vi "UI CMD HOLDER.vi"(8 "error in (no error)":errorcluster, 10 "VI in":refnum<vi>, 11 "Stop Event":refnum<user-event>) -> (0 "error out":errorcluster)   [LabVIEW 2020]
uses:
  PCT FGV CMD.ctl
  Popup/Popup Dialog States.ctl
  Settings/Settings.ctl
  Logging/Save Configuration.ctl
  LOG/LOG Configuration.ctl
  Message Queue/Message Cluster.ctl
  ALARM/ALARM Configuration.ctl
  Valve Control/AM Configuration.ctl
  Test Driver/Test Driver Configuration.ctl
  Test Driver/System Preset.ctl
  Test Driver/Test Type.ctl
  Report/REP Configuration.ctl
  Report/Test Setting.ctl
  MOTOR/PS Hardware Configuration.ctl
  DMM/PalmSense Hardware Configuration.ctl
  <instrlib>/PalmSens SDK for LabVIEW 5.10/PalmSens/PalmSens.lvclass
  Hiden Scanner/Scanner Hardware Configuration.ctl
  MRC/MRC Configuration.ctl
  WM Pump/Pump Hardware Configuration.ctl
  controls/PCT_UI State.ctl
  Main Menu Selector.ctl
  <vilib>/Utility/miscctls.llb/LVRowAndColumnTypeDef.ctl
  HW Message Cluster.ctl
  REF Single  Name to ref convert.vi
  Message Queue/Enqueue Message (Single).vi
  REFs Name to ref convert.vi
  Message Queue/Enqueue Message (Array).vi
  <vilib>/Utility/error.llb/Error Cluster From Error Code.vi
  <vilib>/ErrorRing/Error Ring.xnode
  Settings/Settings.lvlib
  Message Queue/Message Queue.lvlib
  Settings/Settings Dialog.vi
  User Event - Stop/User Event - Stop.lvlib
  Logging/SAVE.lvlib
  LOG/LOG.lvlib
  ALARM/QCT ALARM.lvlib
  Popup/Popup Dialog.lvlib
  Report/Report.lvlib
  Settings/HW Configuration Dialog.vi
  MOTOR/MOTOR.lvlib
  Test Driver/Test Driver.lvlib
  Motion/Motion.lvlib
  DMM/PalmSens.lvlib
  Hiden Scanner/Hiden Scanner.lvlib
  Valve Control/Valve Control.lvlib
  MRC/MRC Module.lvlib
  <vilib>/Utility/cursorutil.llb/Set Cursor (Icon Pict).vi
  WM Pump/Pump.lvlib
panel:
  # "UI CMD HOLDER"
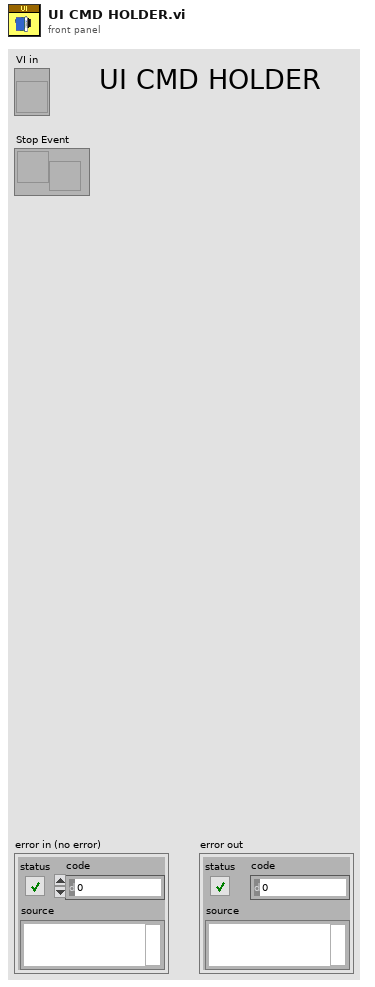
[diagram p1: front panel]
types:
  T1 = typedef "PCT FGV CMD.ctl" = enum16{"INIT", "GET", "SET"}
  T2 = typedef "Message Queue.lvlib/All Message Queues.ctl" = cluster{"UI":refnum<queue>, "Logging":refnum<queue>, "LOG":refnum<queue>, "ALARM":refnum<queue>, "Test":refnum<queue>, "Answer":refnum<queue>, "PLC":refnum<queue>, "DB":refnum<queue>, "Report":refnum<queue>, "OPC":refnum<queue>, "Procedure":refnum<queue>, "PalmSens":refnum<queue>, "SYS 7000 Reader":refnum<queue>, "SWITCH":refnum<queue>, "MOTOR":refnum<queue>, "MOTION":refnum<queue>, "HIDEN":refnum<queue>, "VALVE":refnum<queue>, "MFC":refnum<queue>, "PUMP IN":refnum<queue>, "PUMP OUT":refnum<queue>}
  T3 = typedef "PCT Data REFs.ctl" = cluster{"PLC AI Notifier":refnum<notifier>, "PS Data Queue":refnum<queue>, "BTN Queue":refnum<queue>, "PLC DI notifier":refnum<notifier>, "Timer notifier":refnum<notifier>, "DMM PS":refnum<notifier>, "DMM Gages":refnum<notifier>, "XYZ notifier":refnum<notifier>, "Test Notifier":refnum<notifier>, "Scanner notifier":refnum<notifier>, "OPC Notifier":refnum<notifier>, "HIDEN queue":refnum<queue>}
  T4 = cluster{"Type CMD":string, "Mode CMD":string, "Main CMD":string}
  T5 = typedef "Popup Dialog.lvlib/Popup Dialog States.ctl" = enum32{"Complete", "Failed", "Preparing", "Stopping", "Error", "Saved", "Saving", "Closing"}
  T6 = typedef "PCT_UI State.ctl" = enum16{"Idle", "Procedure Started", "Procedure Paused"}
  T7 = typedef "Settings.lvlib/Settings.ctl" = cluster{"Support":cluster{"Save Configuration":T8, "LOG Configuration":T9, "ALARM Configuration":T10, "User Details":string[], "Radome Type":string, "Timer Configuration":T11}, "Process":cluster{"Test Configuration":T12}, "Report Configuration":T15, "History Data":cluster{"Tests":string[][], "Test Name":string}, "Motor Configuration":T17, "PalmSense  Configuration":T18, "Hiden Scanner Resources":T19, "MFC Configuration":T20, "Pump Configuration":T21}
  T8 = typedef "SAVE.lvlib/Save Configuration.ctl" = cluster{"Log File Base Path":path, "TDMS File Reference":refnum<k34>, "Reset":bool, "Wait":dbl, "Start Time":dbl, "Update Rate":u16, "Channel Names":string[], "System Preset":variant}
  T9 = typedef "LOG.lvlib/LOG Configuration.ctl" = cluster{"LOG REF":refnum<vi>, "Writer Queue":refnum<queue>, "Log Path":path, "LOG":bool}
  T10 = typedef "QCT ALARM.lvlib/ALARM Configuration.ctl" = cluster{"LOG REF":refnum<vi>, "Writer Queue":refnum<queue>, "Log Path":path, "UPS standby":bool, "status code":i32, "SP":dbl[], "Over Sens Status":dbl[]}
  T11 = typedef "Valve Control.lvlib/AM Configuration.ctl" = cluster{"Wait":dbl, "Next Step":string, "Writer Queue":refnum<queue>, "Reset":bool, "VISA resource":refnum<visa-resource-name>, "Status":bool[], "Valve Time":dbl[], "Timer queue":refnum<queue>, "Current valve":i32, "Enable":bool}
  T12 = typedef "Test Driver.lvlib/Test Driver Configuration.ctl" = cluster{"current Step":i32, "Wait":dbl, "Next Step":string, "Writer Queue":refnum<queue>, "Reset":bool, "SEQ Time":i32, "General Reset":bool, "Cycles":i32, "Status":bool[], "Ready":bool[], "Backward":bool, "Current SP":dbl[], "System Preset":T13, "Test Type":T14, "Sample Count":i32, "Local Queues":cluster{"Cycles queue":refnum<queue>, "Step queue":refnum<queue>, "RES Queue":refnum<queue>, "Clean queue":refnum<queue>, "PS Scan queue":refnum<queue>}, "current Clean":i32, "PS Measure Plan":u16[]}
  T13 = typedef "System Preset.ctl" = cluster{"Test Configuration":cluster{"Cycles":i32, "Z Up":dbl, "SP List":dbl[][], "Operator":string, "Point Delay":i32, "Z Up 2":dbl, "Cleaning In":dbl, "Cleaning Out":dbl, "Cleaning Cycles":i32}, "Test_Start_date":string}
  T14 = typedef "Test Driver.lvlib/Test Type.ctl" = enum16{"Calibration", "Test"}
  T15 = typedef "Report.lvlib/REP Configuration.ctl" = cluster{"Test Setting":T16, "Measurements":string[][], "LOG REF":refnum<vi>, "Report Template":path, "Save Report path":path, "Data File Path":path, "Popup Dialog":bool}
  T16 = typedef "Report.lvlib/Test Setting.ctl" = cluster{"Test_Num":i32, "Test_ID":i32, "Proc_ID":i32, "Max Force":dbl, "User":string, "SN":string, "Date":string}
  T17 = typedef "MOTOR.lvlib/PS Hardware Configuration.ctl" = cluster{"Tango HW":cluster{"VISA resource":refnum<visa-resource-name>, "Baud Rate (115200)":i32, "lAnInterfaceType":i32, "bAShowProt":i32}, "Writer Queue":refnum<queue>, "Status":bool, "Abs Position":i32[], "Axis Velocity":cluster{"dX":dbl, "dY":dbl, "dZ":dbl, "dA":dbl}, "acceleration ":dbl, "Z direction":enum16{"Up", "Down"}, "Position Mode":string, "plLSID":i32}
  T18 = typedef "PalmSens.lvlib/PalmSense Hardware Configuration.ctl" = cluster{"PalmSens.lvclass":refnum<class "PalmSens.lvclass">, "Writer Queue":refnum<queue>, "Enable":bool, "Is Measuring Ref":refnum<vi>, "Method":cluster{"Name":string, "Method Ref":variant}, "PS Live Curve Result":refnum<vi>}
  T19 = typedef "Hiden Scanner.lvlib/Scanner Hardware Configuration.ctl" = cluster{"Link":cluster{"Connection":enum16{"Serial", "TCP/IP", "USB"}, "Host or IP address (TCP/IP)":string, "Port (Serial/USB)":string}, "VISA resource":refnum<visa-resource-name>, "Writer Queue":refnum<queue>, "Status":bool}
  T20 = typedef "MRC Module.lvlib/MRC Configuration.ctl" = cluster{"MFC Definition":cluster{"MFC Port":refnum<visa-resource-name>, "MFC Enable":bool, "Baud Rate":i32, "Interface type":enum32{"RS-485", "RS-232"}, "Address":i32}, "Set Point Options":cluster{"Setpoint Value":dbl, "Mass Flow EU 2":string, "Setpoint Source":string, "Valve Mode":string}, "Writer Queue":refnum<queue>, "Enable":bool, "Update Rate":u32, "MRC Chamber Enable":bool, "Selected Gas":string, "Address String":string}
  T21 = typedef "Pump.lvlib/Pump Hardware Configuration.ctl" = cluster{"Pump  name":refnum<visa-resource-name>[], "Writer Queue":refnum<queue>, "Pump Info":cluster{"Pump Type":string, "Speed":i32, "Direction":u16, "Running":bool}, "Current Pump Name":refnum<visa-resource-name>, "Wait":dbl, "Next Step":string, "Reset":bool}
  T22 = enum16{"open", "open or create", "create or replace", "create", "open (read-only)"}
  T23 = typedef "Main Menu Selector.ctl" = enum16{"Main Screen", "Test Setting", "Calibration", "History", "Admin", "Switch User", "About", "Exit"}
  T24 = cluster{"Back-Front Switch":bool, "NewVal":enum32{"1", "2", "3", "4", "5", "6", "7", "8", "9", "10", "11", "12", "13", "14", "15", "16", "17", "18", "19", "20"}}
  T25 = cluster{"Writer Queue":refnum<queue>, "Timeout":dbl[], "Status":bool[]}
  T26 = enum16{"isDO_Section_0", "isDO_Section_90", "isDO_Section_180", "isDO_Section_270", "Mode", "Start", "Reset_Error", "Heart_Beat", "Polling_Cylinder", "Turning_Cylinder", "Locking_Cylinder"}
  T27 = cluster{"Channels":enum16{"isDO_Section_0", "isDO_Section_90", "isDO_Section_180", "isDO_Section_270", "Mode", "Start", "Reset_Error", "Heart_Beat", "Polling_Cylinder", "Turning_Cylinder", "Locking_Cylinder"}, "Status":bool}
  T28 = cluster{"register":dbl, "register":dbl, "register":dbl, "register":dbl}[]
  T29 = typedef "Message Queue.lvlib/Message Cluster.ctl" = cluster{"Message":string, "Message Data":variant}
  T30 = typedef "LVRowAndColumnTypeDef.ctl" = cluster{"Row":i32, "Column":i32}
  T31 = typedef "Message Queue.lvlib/HW Message Cluster.ctl" = cluster{"Writer Queue":refnum<queue>, "Writer Data":T29}
  T32 = enum32{"1", "2", "3", "4", "5", "6", "7", "8", "9", "10", "11", "12", "13", "14", "15", "16", "17", "18", "19", "20"}
  T33 = cluster{"Pump Type":string, "Speed":i32, "Direction":u16, "Running":bool}
  T34 = cluster{"Current SP[0]":dbl, "Current SP[1]":dbl}
  T35 = cluster{"Current SP[0]":i32, "Current SP[1]":i32}
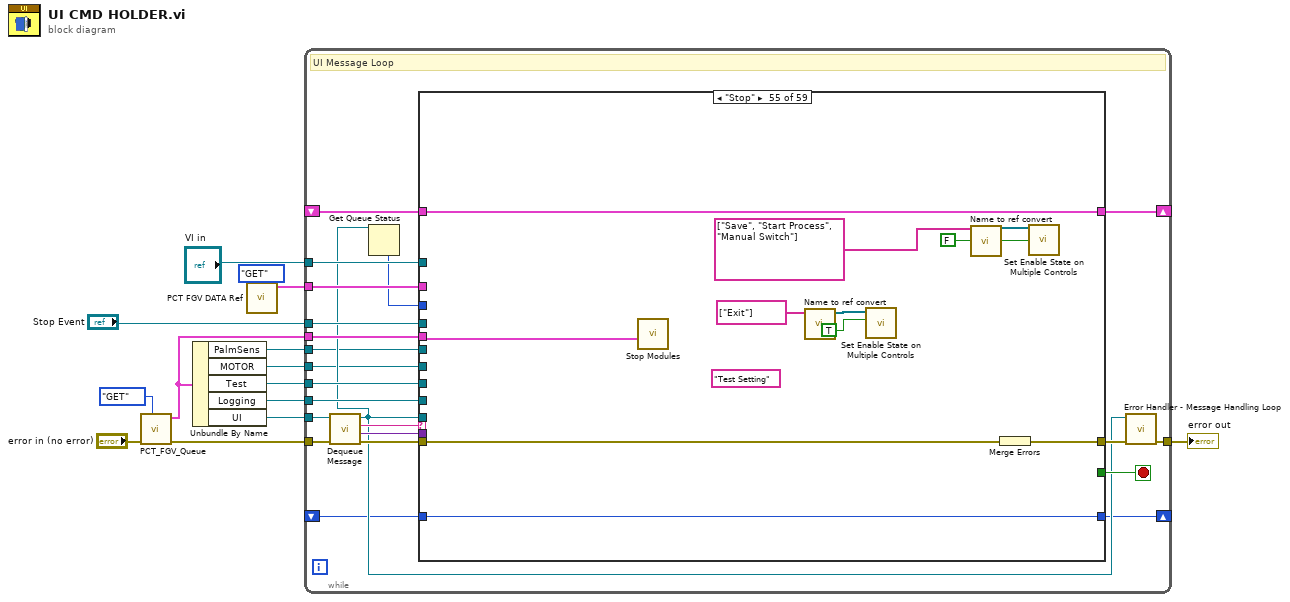
[diagram p0: block diagram]
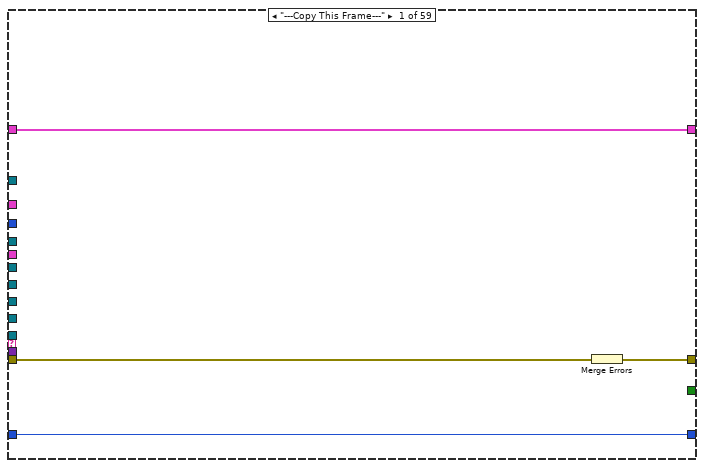
[diagram p2: hidden frame]
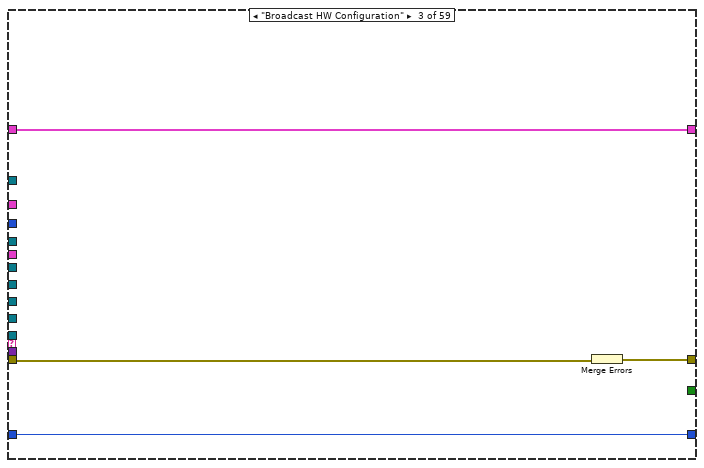
[diagram p4: hidden frame]
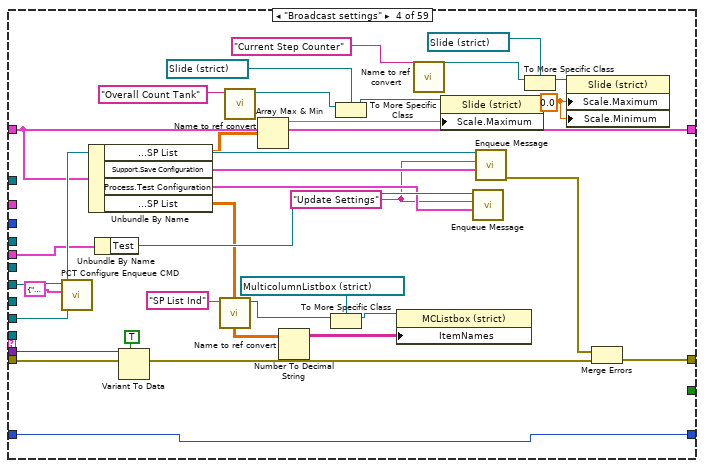
[diagram p5: hidden frame]
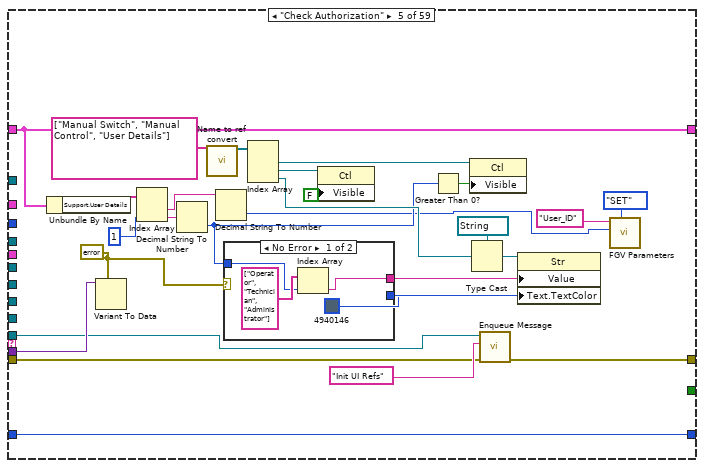
[diagram p6: hidden frame]
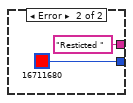
[diagram p7: hidden frame]
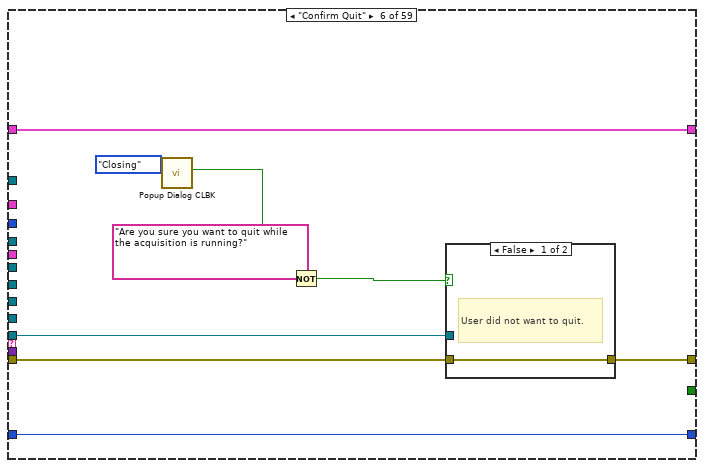
[diagram p8: hidden frame]
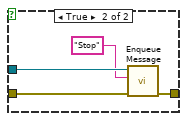
[diagram p9: hidden frame]
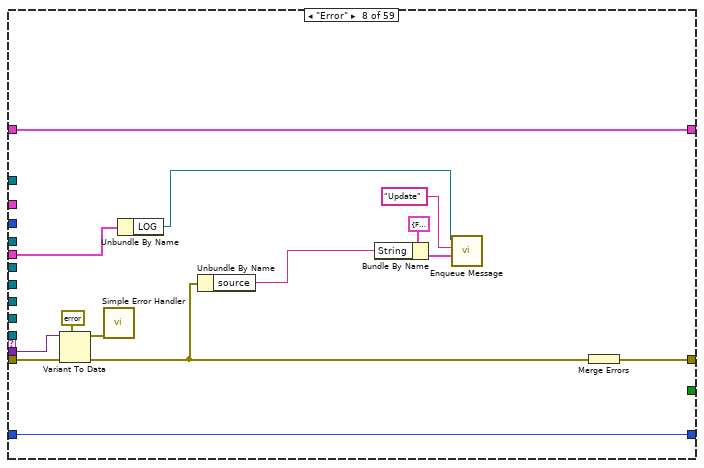
[diagram p11: hidden frame]
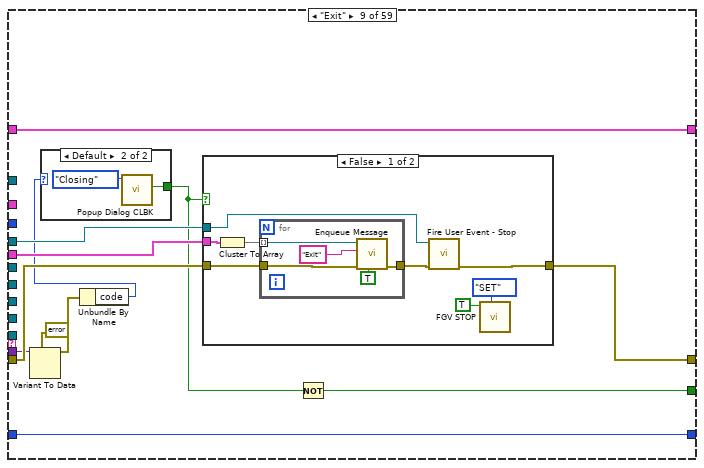
[diagram p12: hidden frame]
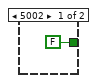
[diagram p13: hidden frame]
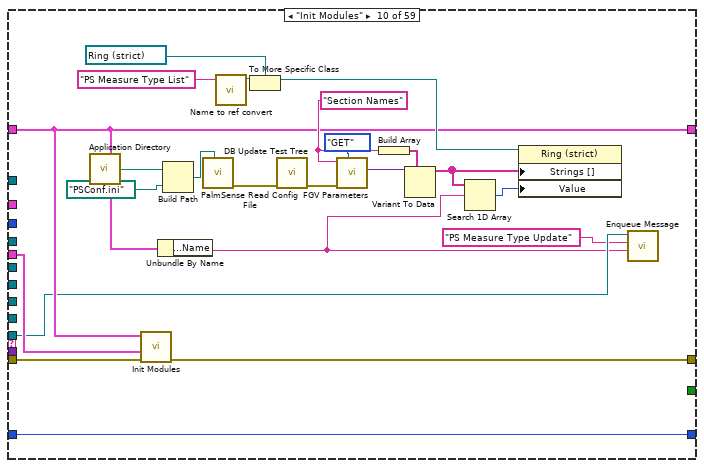
[diagram p15: hidden frame]
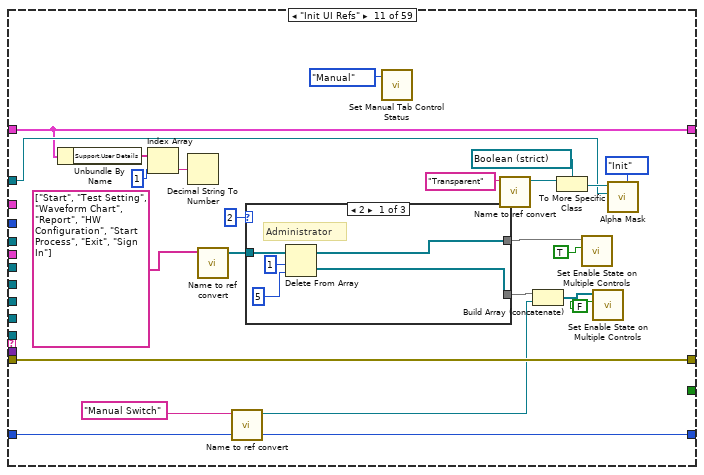
[diagram p16: hidden frame]
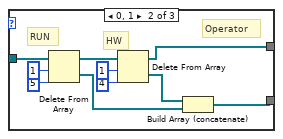
[diagram p17: hidden frame]
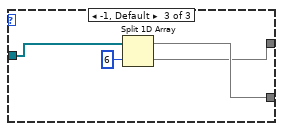
[diagram p18: hidden frame]
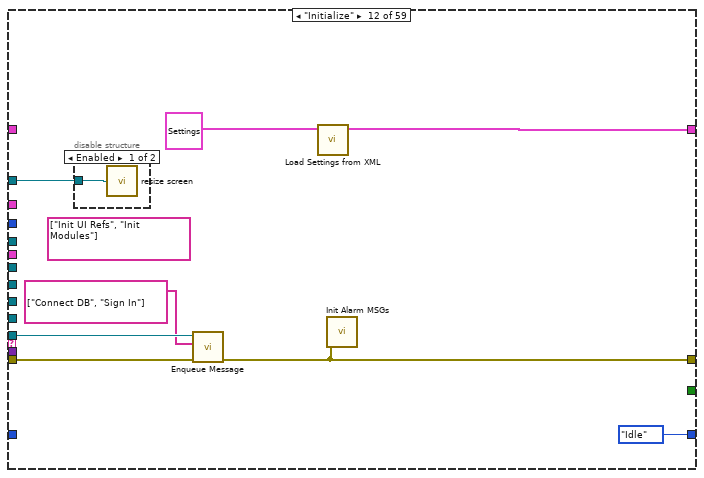
[diagram p19: hidden frame]
diagram:
  n1 = call "PCT_FGV_Queue.vi"("CMD"=PCT_FGV_CMD."GET", "error in (no error)"="error in (no error)") -> ("error out"=w2:errorcluster, "Message Queues out"=w8:T2)  [unwired: 8 in]
  n2 = Unbundle By Name(w8) -> ("PalmSens"=w1:refnum<queue>, "MOTOR"=w3:refnum<queue>, "Test"=w7:refnum<queue>, "Logging"=w12:refnum<queue>, "UI"=w13:refnum<queue>)
  n3 = call "PCT FGV DATA Ref.vi"("CMD"=PCT_FGV_CMD."GET") -> ("Data REF"=w4:T3)  [unwired: 9 in, 1 out]
  n4 = while {
    tunnel: w13 -> [w30]
    tunnel: "Stop Event" -> [w35]
    shift-right: [w29] -> _
    shift-left: _ -> [w28]
    tunnel: w12 -> [w27]
    tunnel: w2 -> [w34]
    tunnel: [w26] -> w14
    tunnel: w8 -> [w24]
    tunnel: w7 -> [w23]
    tunnel: "VI in" -> [w22]
    tunnel: w4 -> [w21]
    tunnel: w3 -> [w18]
    shift-right: [w17] -> _
    shift-left: _ -> [w16]
    tunnel: w1 -> [w15]
    stop <- w36 stop-if-true
    # "UI Message Loop"
    n5 = call "Dequeue Message.vi"("error in (no error)"=w34, "Message Queue"=w30) -> ("error out"=w33:errorcluster, "Message Data"=w31:variant, "Message"=w32:string, "dup Message Queue"=w20:refnum<queue>)  [unwired: 6 in]
    n6 = Get Queue Status(queue=w20) -> (# elements in queue=w19:i32)  [unwired: 2 in, 7 out]
    n7 = case "Message Cases" shown="\"Stop\"" w32 {
      selector: w32 -> [_ _ _ _ _ _ _ _ _ _ _ _ _ _ _ _ _ _ _ _ _ _ _ _ _ _ _ _ _ _ _ _ _ _ _ w643 _ _ _ _ _ _ _ _ _ _ _ _ _ _ _ _ _ _ _ _ _ _ w1225]
      tunnel: w20 -> [_ _ _ _ w89 w119 _ _ _ w180 _ w244 w256 w283 _ _ _ _ w368 w385 _ w430 _ _ _ _ _ _ _ _ _ w602 _ _ _ _ _ _ _ _ _ _ _ _ _ _ _ _ w782 _ _ w864 _ _ _ _ w937 _ _]
      tunnel: w33 -> [w40 w42 w46 w77 w87 w118 w127 w137 w151 w193 w217 w243 w258 w285 w307 w351 w364 w366 w374 w397 w418 _ w446 w455 w467 w496 w509 w546 w568 w574 w583 w606 w612 _ w630 w654 w661 w667 w673 w679 w692 w701 w718 w738 w741 w744 w758 w769 w778 w799 w850 w863 _ w907 w919 w930 w945 w1222 _]
      tunnel: [w39 w42 w47 w79 w86 w117 w127 w139 w153 w191 w217 w239 w254 w281 w306 w351 w361 w366 w375 w397 w418 w423 w446 w455 w467 w496 w509 w546 w568 w574 w583 w606 w612 w621 w629 w654 w661 w667 w673 w679 w692 w701 w718 w738 w741 w744 w759 w769 w779 w801 w850 w861 w892 w907 w920 w930 w936 w1222 w1224] -> w25
      tunnel: [_ _ _ _ _ _ _ _ w147 _ _ _ _ _ _ _ _ _ _ _ _ _ _ _ _ _ _ _ _ _ _ _ _ _ _ _ _ _ _ _ _ _ _ _ _ _ _ _ _ _ _ _ _ _ _ _ _ _ _] -> w36
      tunnel: w31 -> [_ _ _ w70 w96 _ _ w140 w150 _ _ _ _ _ w302 _ w360 _ w372 w389 w417 w427 w442 w454 w466 _ w508 _ w564 w573 w581 w604 _ _ w633 w651 w658 w665 w671 w677 w683 w695 w716 w734 _ _ w751 _ _ _ _ _ _ _ _ w928 w944 w1213 _]
      tunnel: w35 -> [_ _ _ _ _ _ _ _ w154 _ _ _ _ _ _ _ _ _ _ _ _ _ _ _ _ _ _ _ _ _ _ _ _ _ _ _ _ _ _ _ _ _ _ _ _ _ _ _ _ _ _ _ _ _ _ _ _ _ _]
      tunnel: [w38 w43 w45 w68 w98 w120 w128 w142 w152 w181 w208 w238 w247 w271 w308 w349 w363 w367 w373 w394 w419 w437 w447 w456 w468 w484 w510 w547 w569 w575 w582 w605 w611 w618 w631 w653 w662 w668 w674 w680 w693 w702 w719 w731 w742 w745 w757 w768 w783 w798 w849 w862 w883 w906 w918 w929 w938 w1221 w1226] -> w29
      tunnel: w28 -> [w38 w43 w45 w68 w98 w120 w128 w142 w152 w181 w208 _ w259 w273 w308 w349 w363 w367 w373 w394 w419 w437 w447 w456 w468 w484 w510 w547 w569 w575 w582 w605 w611 w618 w631 w653 w662 w668 w674 w680 w693 w702 w719 w739 w742 w745 w757 w768 w784 w798 w849 w862 w883 w906 w918 w929 w939 w1221 w1226]
      tunnel: w27 -> [_ _ _ w75 _ _ _ _ _ _ _ _ _ _ _ _ w362 _ _ _ _ _ _ _ _ _ _ _ _ _ _ _ _ _ _ _ _ _ _ _ _ _ _ _ _ _ _ _ _ _ _ _ _ _ _ _ _ _ _]
      tunnel: w24 -> [_ _ _ w67 _ _ _ w132 w149 w194 _ _ _ _ _ _ _ _ _ _ w416 w434 w441 w449 w463 _ _ _ _ _ w578 w600 _ _ _ w647 _ _ _ _ _ _ _ _ _ _ w755 w765 _ _ _ _ w868 _ w914 _ w934 _ _]
      tunnel: w23 -> [_ _ _ _ _ _ _ _ _ _ _ _ _ _ _ _ _ _ _ _ _ _ _ _ _ _ _ _ _ _ _ _ _ w620 _ _ _ _ _ _ _ _ _ _ _ _ _ _ _ w800 _ _ w891 _ _ _ _ _ _]
      tunnel: w22 -> [_ _ _ _ _ _ _ _ _ _ w212 w240 _ _ _ _ _ _ _ _ _ w421 _ _ _ _ _ w514 _ _ _ _ _ _ _ _ _ _ _ _ _ _ _ _ _ _ _ w762 _ _ _ _ _ _ _ _ _ _ _]
      tunnel: w21 -> [_ _ _ _ _ _ _ _ _ _ _ _ _ _ _ _ _ _ _ _ _ w429 _ _ _ w493 _ w544 _ _ _ _ _ _ _ _ _ _ _ _ _ _ _ _ _ _ _ _ _ w795 _ _ _ _ _ _ w935 _ _]
      tunnel: w19 -> [_ _ _ _ _ _ _ _ _ _ _ _ _ _ _ _ _ _ _ _ _ _ _ _ _ _ _ _ _ _ _ _ _ _ _ _ _ _ _ _ _ _ _ _ _ _ _ _ _ _ _ _ _ _ _ _ _ _ _]
      tunnel: w18 -> [_ _ _ w71 _ _ _ _ _ _ _ _ _ _ _ _ _ _ _ w390 _ w436 _ _ w464 _ w506 w511 w566 w572 _ _ w609 _ w623 _ w660 w666 w672 w678 w691 w700 w717 _ _ _ _ w767 _ w796 _ _ w877 _ _ _ w931 _ _]
      tunnel: [w37 w41 w44 w55 w85 w113 w126 w136 w143 w192 w197 PCT_UI_State."Idle" ("UI State") w246 w272 w305 w350 w354 w365 w371 w388 w400 w435 w445 w453 w465 w495 w503 w545 w563 w570 w580 w603 w610 PCT_UI_State."Procedure Paused" ("UI State") w622 w637 w657 w664 w670 w676 w690 w699 w715 w737 w740 w743 w746 w766 w774 w797 w839 w853 PCT_UI_State."Idle" ("UI State") w895 w910 w921 w932 w1220 w1223] -> w17
      tunnel: w16 -> [w37 w41 w44 w55 w85 w113 w126 w136 w143 w192 w197 _ w246 w272 w305 w350 w354 w365 w371 w388 w400 w435 w445 w453 w465 w495 w503 w545 w563 w570 w580 w603 w610 _ w622 w637 w657 w664 w670 w676 w690 w699 w715 w737 w740 w743 w746 w766 w774 w797 w839 w853 _ w895 w910 w921 w933 w1220 w1223]
      tunnel: w15 -> [_ _ _ _ _ _ _ _ _ _ _ _ _ _ _ _ _ _ _ _ _ _ _ _ _ w494 _ _ _ _ _ _ _ _ _ _ _ _ _ _ _ _ _ _ _ _ _ _ _ _ _ _ _ _ _ _ _ _ _]
      frame "---Copy This Frame---" {
        # "Duplicate this frame when creating new messages.  Change this comment in the duplicated frame to describe this message."
        n8 = Merge Errors(w40) -> (w39:errorcluster)
      }
      frame "Acquisition Stopped" {
        # "Logic for determining what action to take when the acquisition has stopped."
      }
      frame "Broadcast HW Configuration" {
        # "Broadcast settings - Send the 'Update Settings' message to the Logging and Acquisition message loops."
        n9 = Merge Errors(w46) -> (w47:errorcluster)
      }
      frame "Broadcast settings" {
        w56 = 0.0 ("Scale.Range:Maximum")
        w54 = "Update Settings" ("Message")
        # "Broadcast settings - Send the 'Update Settings' message to the Logging and Acquisition message loops."
        n10 = call "PCT Configure Enqueue CMD.vi"("CMD"=T4 {"Type CMD"="SP", "Mode CMD"="", "Main CMD"="Configure"}, "CMD Queue in"=w71) -> ()  [unwired: 7 in, 3 out]
        n11 = Unbundle By Name(w68) -> ("Process.Test Configuration.System Preset.Test Configuration.SP List"=w62:dbl[][], "Support.Save Configuration"=w76:T8, "Process.Test Configuration"=w73:T12, "Process.Test Configuration.System Preset.Test Configuration.SP List"=w50:dbl[][])
        n12 = Unbundle By Name(w67) -> ("Test"=w74:refnum<queue>)
        n13 = Variant To Data(type=TRUE, Variant=w70) -> ()  [unwired: 1 in, 2 out]
        n14 = call-poly "Name to ref convert.vi"("name"="SP List Ind") -> ("First REF"=w52:refnum<vi>)  [unwired: 10 in]
        n15 = call-poly "Name to ref convert.vi"("name"="Overall Count Tank") -> ("First REF"=w65:refnum<vi>)  [unwired: 10 in]
        n16 = Array Max & Min(array=w62) -> (max value=w61:dbl)  [unwired: 3 out]
        n17 = Number To Decimal String(number=w50) -> (decimal integer string=w49:string[][])  [unwired: 1 in]
        n18 = To More Specific Class(target class=refnum<vi> refnum ("SP List Ind"), reference=w52) -> (specific class reference=w51:refnum<vi>)  [unwired: 1 in, 1 out]
        n19 = To More Specific Class(target class=refnum<vi> refnum ("Overall Count Tank"), reference=w65) -> (specific class reference=w63:refnum<vi>)  [unwired: 1 in, 1 out]
        n20 = property class="MCListbox (strict)"(reference=w51, "ItemNames"=w49) -> ()  [unwired: 1 in, 2 out]
        n21 = call-poly "Name to ref convert.vi"("name"="Current Step Counter") -> ("First REF"=w59:refnum<vi>)  [unwired: 10 in]
        n22 = property class="Slide (strict)"(reference=w63, "Scale.Maximum"=w61) -> ()  [unwired: 1 in, 2 out]
        n23 = call-poly "Enqueue Message.vi"("Message Data"=w73, "Message"=w54, "Message Queue"=w74) -> ()  [unwired: 7 in, 2 out]
        n24 = call-poly "Enqueue Message.vi"("Message Data"=w76, "Message"=w54, "Message Queue"=w75) -> ("error out"=w78:errorcluster)  [unwired: 7 in, 1 out]
        n25 = To More Specific Class(target class=refnum<vi> refnum ("Overall Count Tank"), reference=w59) -> (specific class reference=w57:refnum<vi>)  [unwired: 1 in, 1 out]
        n26 = property class="Slide (strict)"(reference=w57, "Scale.Maximum"=w56, "Scale.Minimum"=w56) -> ()  [unwired: 1 in, 2 out]
        n27 = Merge Errors(w78, w77) -> (w79:errorcluster)
      }
      frame "Check Authorization" {
        w80 = errorcluster {"status"=FALSE, "code"=0, "source"=""} ("error out")
        n28 = Unbundle By Name(w98) -> ("Support.User Details"=w97:string[])
        n29 = Variant To Data(type=w80, Variant=w96) -> ()  [unwired: 1 in, 2 out]
        n30 = Index Array(array=w97, index #2=1 ("index")) -> (element #1=w82:string, element #2=w105:string)  [unwired: 1 in]
        n31 = Decimal String To Number(string=w105) -> (number=w91:i32)  [unwired: 2 in, 1 out]
        n32 = call-poly "Name to ref convert.vi"("Array in"=string[] ["Manual Switch", "Manual Control", "User Details"] ("name")) -> ("Array out"=w104:refnum<vi>[])  [unwired: 10 in]
        n33 = Decimal String To Number(string=w82) -> (number=w81:i32)  [unwired: 2 in, 1 out]
        n34 = case shown="No Error" w80 {
          tunnel: [w108 "Resticted " ("name")] -> w92
          tunnel: w91 -> [w109 _]
          tunnel: [u32 4940146 u32 16711680] -> w90
          frame No Error {
            n35 = Index Array(array=string[] ["Operator", "Technician", "Administrator"], index=w109) -> (element=w108:string)
          }
          frame Error {
          }
        }
        n36 = Index Array(array=w104) -> (element #1=w102:refnum<vi>, element #2=w100:refnum<vi>, element #3=w95:refnum<vi>)  [unwired: 3 in]
        n37 = property class="Ctl"(reference=w100, "Visible"=FALSE) -> ()  [unwired: 1 in, 2 out]
        n38 = Greater Than 0?(x=w91) -> (x > 0?=w101:bool)
        n39 = property class="Ctl"(reference=w102, "Visible"=w101) -> ()  [unwired: 1 in, 2 out]
        n40 = Type Cast(type=refnum<vi> refnum ("LOG"), x=w95) -> (*(type *) &x=w93:refnum<vi>)
        n41 = call-poly "Enqueue Message.vi"("error in (no error)"=w87, "Message"="Init UI Refs" ("name"), "Message Queue"=w89) -> ("error out"=w86:errorcluster)  [unwired: 7 in, 1 out]
        n42 = property class="Str"(reference=w93, "Value"=w92, "Text.TextColor"=w90) -> ()  [unwired: 1 in, 2 out]
        n43 = call "FGV Parameters.vi"("CMD"=PCT_FGV_CMD."SET", "input"=w81, "Key"="User_ID") -> ()  [unwired: 6 in, 3 out]
      }
      frame "Confirm Quit" {
        (unwired) "Are you sure you want to quit while the acquisition is running?" ("Confirm Quit Message")
        # "Confirm Quit - Message that can confirm whether or not the user wants to exit the application."
        n44 = call "Popup Dialog CLBK.vi"("Tab Control"=Popup_Dialog_States."Closing") -> ("canceled?"=w115:bool)  [unwired: 8 in, 2 out]
        n45 = Not(x=w115) -> (.not. x?=w114:bool)
        n46 = case shown="False" w114 {
          tunnel: w119 -> [_ w124]
          tunnel: w118 -> [w121 w125]
          tunnel: [w121 w123] -> w117
          frame False {
            # "User did not want to quit."
          }
          frame True {
            n47 = call-poly "Enqueue Message.vi"("error in (no error)"=w125, "Message"="Stop", "Message Queue"=w124) -> ("error out"=w123:errorcluster)  [unwired: 7 in, 1 out]
          }
        }
      }
      frame "Connect DB" {
      }
      frame "Error" {
        # "Error - Display an error dialog. This message is sent by the \"Error Handler\" VIs at the end of other loops in this application."
        n48 = Variant To Data(error in=w137, type=errorcluster {"status"=FALSE, "code"=0, "source"=""} ("error constant"), Variant=w140) -> (data=w138:errorcluster, error out=w130:errorcluster)
        n49 = call <vilib>:"Simple Error Handler.vi"("error in (no error)"=w138) -> ()  [unwired: 4 in, 5 out]
        n50 = Unbundle By Name(w132) -> ("LOG"=w131:refnum<queue>)
        n51 = Unbundle By Name(w130) -> ("source"=w129:string)
        n52 = Bundle By Name(cluster=cluster{"Replace":bool, "String":string} {"Replace"=FALSE, "String"="Procedure was started"}, "String"=w129) -> (w133:cluster{"Replace":bool, "String":string})
        n53 = call-poly "Enqueue Message.vi"("Message Data"=w133, "Message"="Update" ("Main CMD"), "Message Queue"=w131) -> ()  [unwired: 7 in, 2 out]
        n54 = Merge Errors(w130) -> (w139:errorcluster)
      }
      frame "Exit" {
        # "Exit - Send Exit messages to the Acquisition and Logging loops, and fire the user event to stop the Event Handling Loop."
        n55 = Variant To Data(type=errorcluster {"status"=FALSE, "code"=0, "source"=""} ("error constant"), Variant=w150) -> (data=w145:errorcluster)  [unwired: 1 in, 1 out]
        n56 = Unbundle By Name(w145) -> ("code"=w144:i32)
        n57 = case shown="Default" w144 {
          tunnel: [FALSE ("canceled?") w156] -> w148
          frame 5002 {
          }
          frame Default {
            n58 = call "Popup Dialog CLBK.vi"("Tab Control"=Popup_Dialog_States."Closing") -> ("canceled?"=w156:bool)  [unwired: 8 in, 2 out]
          }
        }
        n59 = case shown="False" w148 {
          tunnel: w154 -> [w165 _]
          tunnel: [w164 w171] -> w153
          tunnel: w151 -> [w163 w171]
          tunnel: w149 -> [w161 _]
          frame False {
            n60 = Cluster To Array(cluster=w161) -> (array=w160:refnum<queue>[])
            n61 = for {
              tunnel: w160 -> [w170] mode=indexing
              tunnel: w163 -> [w167]
              tunnel: [w166] -> w162
              n62 = call-poly "Enqueue Message.vi"("Priority Message? (F)"=TRUE, "error in (no error)"=w167, "Message"="Exit", "Message Queue"=w170) -> ("error out"=w166:errorcluster)  [unwired: 6 in, 1 out]
            }
            n63 = call "Fire User Event - Stop.vi"("error in (no error)"=w162, "User Event - Stop"=w165) -> ("error out"=w164:errorcluster)  [unwired: 9 in]
            n64 = call "FGV STOP.vi"("CMD"=PCT_FGV_CMD."SET", "input"=TRUE) -> ()  [unwired: 8 in, 2 out]
          }
          frame True {
          }
        }
        n65 = Not(x=w148) -> (.not. x?=w147:bool)
      }
      frame "Init Modules" {
        w188 = "Section Names"
        # "Init UI Refs - Store control references for UI controls.  Also enable/disable controls appropriately."
        n66 = call <vilib>:"Application Directory.vi"() -> ("Application Directory"=w174:path)
        n67 = call "Init Modules.vi"("error in (no error)"=w193, "Message Queues in"=w194, "Settings"=w181) -> ("error out"=w191:errorcluster)  [unwired: 8 in]
        n68 = Unbundle By Name(w181) -> ("PalmSense  Configuration.Method.Name"=w176:string)
        n69 = Build Path(base path=w174, name or relative path=path "PSConf.ini" ("configuration file path")) -> (appended path=w172:path)
        n70 = call "PalmSense Read Config File.vi"("configuration file path"=w172) -> ("error out"=w190:errorcluster)  [unwired: 10 in]
        n71 = call-poly "Name to ref convert.vi"("name"="PS Measure Type List") -> ("First REF"=w185:refnum<vi>)  [unwired: 10 in]
        n72 = To More Specific Class(target class=refnum<vi> refnum ("PS Measure Type List"), reference=w185) -> (specific class reference=w182:refnum<vi>)  [unwired: 1 in, 1 out]
        n73 = call "DB Update Test Tree.vi"("error in (no error)"=w190) -> ("error out"=w186:errorcluster)  [unwired: 10 in]
        n74 = call "FGV Parameters.vi"("CMD"=PCT_FGV_CMD."GET", "error in (no error)"=w186, "Key"=w188) -> ("output"=w178:variant)  [unwired: 6 in, 2 out]
        n75 = Build Array(w188) -> (w187:string[])
        n76 = Variant To Data(type=w187, Variant=w178) -> (data=w177:string[])  [unwired: 1 in, 1 out]
        n77 = Search 1D Array(1D array=w177, element=w176) -> (index of element=w175:i32)  [unwired: 1 in]
        n78 = property on="Property Node" class="Ring (strict)"(reference=w182, "Strings []"=w177, "Value"=w175) -> ()  [unwired: 1 in, 2 out]
        n79 = call-poly "Enqueue Message.vi"("Message Data"=w176, "Message"="PS Measure Type Update", "Message Queue"=w180) -> ()  [unwired: 7 in, 2 out]
      }
      frame "Init UI Refs" {
        # "Init UI Refs - Store control references for UI controls.  Also enable/disable controls appropriately."
        n80 = Unbundle By Name(w208) -> ("Support.User Details"=w209:string[])
        n81 = Index Array(array=w209, index=1) -> (element=w210:string)
        n82 = Decimal String To Number(string=w210) -> ()  [unwired: 2 in, 2 out]
        n83 = call-poly "Name to ref convert.vi"("Array in"=string[] ["Start", "Test Setting", "Waveform Chart", "Report", "HW Configuration", "Start Process", "Exit", "Sign In"]) -> ("Array out"=w207:refnum<vi>[])  [unwired: 10 in]
        n84 = call-poly "Name to ref convert.vi"("name"="Manual Switch") -> ("First REF"=w198:refnum<vi>)  [unwired: 10 in]
        n85 = case shown="2" 2 {
          tunnel: w207 -> [w222 w232 w236]
          tunnel: [w218 w224 w234] -> w204
          tunnel: [w219 w223 w233] -> w203
          frame 2 {
            # "Administrator"
            n86 = Delete From Array(array=w222, length=1, index=5) -> (deleted portion=w218:refnum<vi>[], array with subset deleted=w219:refnum<vi>[])
          }
          frame 0, 1 {
            # "HW"
            # "RUN"
            # "Operator"
            n87 = Delete From Array(array=w232, length=1, index=5) -> (deleted portion=w226:refnum<vi>[], array with subset deleted=w227:refnum<vi>[])
            n88 = Delete From Array(array=w227, length=1, index=4) -> (deleted portion=w225:refnum<vi>[], array with subset deleted=w223:refnum<vi>[])
            n89 = Build Array (concatenate)(w225, w226) -> (w224:refnum<vi>[])
          }
          frame -1, Default {
            n90 = Split 1D Array(array=w236, index=6) -> (first subarray=w234:refnum<vi>[], second subarray=w233:refnum<vi>[])
          }
        }
        n91 = call "Set Manual Tab Control Status.vi"("Value"=enum32{"Manual", "Test"}."Manual") -> ()  [unwired: 11 in]
        n92 = call-poly "Name to ref convert.vi"("name"="Transparent") -> ("First REF"=w201:refnum<vi>)  [unwired: 10 in]
        n93 = Build Array (concatenate)(w204, w198) -> (w199:refnum<vi>[])
        n94 = To More Specific Class(target class=refnum<vi> refnum ("Button Ref"), reference=w201) -> (specific class reference=w215:refnum<vi>)  [unwired: 1 in, 1 out]
        n95 = call "Set Enable State on Multiple Controls.vi"("Enable?"=TRUE, "Controls"=w203) -> ()  [unwired: 9 in, 1 out]
        n96 = call "Set Enable State on Multiple Controls.vi"("Enable?"=FALSE, "Controls"=w199) -> ()  [unwired: 9 in, 1 out]
        n97 = call "Alpha Mask.vi"("State"=enum16{"Init", "Open", "Close"}."Init", "This VI"=w212, "Button Ref"=w215) -> ()  [unwired: 7 in, 2 out]
      }
      frame "Initialize" {
        (unwired) string[] ["Init UI Refs", "Init Modules"]
        # "Initialize - Get configuration settings, then message the UI to initialize, and broadcast the settings to the other message loops."
        n98 = disable-structure shown="Enabled" {
          disable-tunnel: w240 -> [w245 _]
          frame Enabled {
            n99 = call "resize screen.vi"("This VI"=w245) -> ()
          }
          frame Disabled {
          }
        }
        n100 = call-poly "Enqueue Message.vi"("error in (no error)"=w243, "Message Array"=string[] ["Connect DB", "Sign In"], "Message Queue"=w244) -> ("error out"=w239:errorcluster)  [unwired: 7 in, 1 out]
        n101 = call "Load Settings from XML.vi"("Settings in"=T7 {"Support"={"Save Configuration"={"Log File Base Path"=path "", "TDMS File Reference"=refnum, "Reset"=FALSE, "Wait"=0.0, "Start Time"=0.0, "Update Rate"=1, "Channel Names"=[], "System Preset"=variant}, "LOG Configuration"={"LOG REF"=refnum, "Writer Queue"=refnum, "Log Path"=path "", "LOG"=FALSE}, "ALARM Configuration"={"LOG REF"=refnum, "Writer Queue"=refnum, "Log Path"=path "", "UPS standby"=FALSE, "status code"=5001, "SP"=[], "Over Sens Status"=[]}, "User Details"=[], "Radome Type"="", "Timer Configuration"={"Wait"=0.0, "Next Step"="", "Writer Queue"=refnum, "Reset"=FALSE, "VISA resource"="", "Status"=[], "Valve Time"=[], "Timer queue"=refnum, "Current valve"=0, "Enable"=FALSE}}, "Process"={"Test Configuration"={"current Step"=0, "Wait"=0.0, "Next Step"="", "Writer Queue"=refnum, "Reset"=FALSE, "SEQ Time"=0, "General Reset"=FALSE, "Cycles"=0, "Status"=[], "Ready"=[], "Backward"=FALSE, "Current SP"=[], "System Preset"={"Test Configuration"={"Cycles"=0, "Z Up"=0.0, "SP List"=[], "Operator"="", "Point Delay"=0, "Z Up 2"=0.0, "Cleaning In"=0.0, "Cleaning Out"=0.0, "Cleaning Cycles"=0}, "Test_Start_date"=""}, "Test Type"=enum."Calibration", "Sample Count"=0, "Local Queues"={"Cycles queue"=refnum, "Step queue"=refnum, "RES Queue"=refnum, "Clean queue"=refnum, "PS Scan queue"=refnum}, "current Clean"=0, "PS Measure Plan"=[]}}, "Report Configuration"={"Test Setting"={"Test_Num"=0, "Test_ID"=0, "Proc_ID"=0, "Max Force"=0.0, "User"="", "SN"="", "Date"=""}, "Measurements"=[], "LOG REF"=refnum, "Report Template"=path "", "Save Report path"=path "", "Data File Path"=path "", "Popup Dialog"=FALSE}, "History Data"={"Tests"=[], "Test Name"=""}, "Motor Configuration"={"Tango HW"={"VISA resource"="", "Baud Rate (115200)"=2, "lAnInterfaceType"=0, "bAShowProt"=15}, "Writer Queue"=refnum, "Status"=FALSE, "Abs Position"=[], "Axis Velocity"={"dX"=0.0, "dY"=0.0, "dZ"=0.0, "dA"=0.0}, "acceleration "=0.0, "Z direction"=enum."Up", "Position Mode"="", "plLSID"=0}, "PalmSense  Configuration"={"PalmSens.lvclass"=refnum, "Writer Queue"=refnum, "Enable"=FALSE, "Is Measuring Ref"=refnum, "Method"={"Name"="", "Method Ref"=variant}, "PS Live Curve Result"=refnum}, "Hiden Scanner Resources"={"Link"={"Connection"=enum."USB", "Host or IP address (TCP/IP)"="", "Port (Serial/USB)"="COM1"}, "VISA resource"="", "Writer Queue"=refnum, "Status"=FALSE}, "MFC Configuration"={"MFC Definition"={"MFC Port"="", "MFC Enable"=TRUE, "Baud Rate"=0, "Interface type"=enum."RS-485", "Address"=0}, "Set Point Options"={"Setpoint Value"=0.0, "Mass Flow EU 2"="", "Setpoint Source"="", "Valve Mode"=""}, "Writer Queue"=refnum, "Enable"=FALSE, "Update Rate"=0, "MRC Chamber Enable"=FALSE, "Selected Gas"="", "Address String"=""}, "Pump Configuration"={"Pump  name"=[], "Writer Queue"=refnum, "Pump Info"={"Pump Type"="", "Speed"=0, "Direction"=0, "Running"=FALSE}, "Current Pump Name"="", "Wait"=0.0, "Next Step"="", "Reset"=FALSE}} ("Config")) -> ("Settings out"=w238:T7)  [unwired: 9 in, 1 out]
        n102 = call "Init Alarm MSGs.vi"("error in (no error)"=w239) -> ()  [unwired: 10 in, 1 out]
      }
      frame "Launch HW Configuration Dialog" {
        # "Launch Settings Dialog - Launch the Settings Dialog when the user clicks the 'Settings' button."
        n103 = call-by-ref "?"("error in (no error)"=w258, "Settings in"=w259) -> ("error out"=w255:errorcluster, "Cancelled?"=w257:bool, "Settings out"=w247:T7)  [unwired: 8 in, 3 out]
        n104 = call "Prepare Version Info.vi"("Settings"=w247) -> ("String"=w250:string)  [unwired: 7 in, 3 out]
        n105 = case shown="False" w257 {
          tunnel: w256 -> [w265 _]
          tunnel: w255 -> [w264 w266]
          tunnel: [w263 w266] -> w254
          frame False {
            n106 = call-poly "Enqueue Message.vi"("error in (no error)"=w264, "Message"="Broadcast HW Configuration", "Message Queue"=w265) -> ("error out"=w263:errorcluster)  [unwired: 7 in, 1 out]
          }
          frame True {
          }
        }
        n107 = call-poly "Name to ref convert.vi"("Array in"=string[] ["info"] ("name")) -> ("Array out"=w248:refnum<vi>[])  [unwired: 10 in]
        n108 = Index Array(array=w248) -> (element #1=w249:refnum<vi>)  [unwired: 2 in, 1 out]
        n109 = Type Cast(type=refnum<vi> refnum ("LOG"), x=w249) -> (*(type *) &x=w252:refnum<vi>)
        n110 = disable-structure shown="Disabled" {
          disable-tunnel: w252 -> [w261 _]
          disable-tunnel: w250 -> [w260 _]
          frame Disabled {
            n111 = property class="Str"(reference=w261, "Value"=w260) -> ()  [unwired: 1 in, 2 out]
          }
          frame Enabled {
          }
        }
      }
      frame "Launch Settings Dialog" {
        # "Launch Settings Dialog - Launch the Settings Dialog when the user clicks the 'Settings' button."
        n112 = call-by-ref "?"("error in (no error)"=w285, "Settings in"=w273) -> ("error out"=w282:errorcluster, "Cancelled?"=w284:bool, "Settings out"=w271:T7)  [unwired: 8 in, 3 out]
        n113 = Unbundle By Name(w271) -> ("Process.Test Configuration.System Preset.Test Configuration.SP List"=w270:dbl[][], "Process.Test Configuration.System Preset.Test Configuration.Z Up"=w267:dbl)  [unwired: 1 out]
        n114 = call "Prepare Version Info.vi"("Settings"=w271) -> ("Enable"=w274:bool, "String"=w277:string)  [unwired: 7 in, 2 out]
        n115 = Array Max & Min(array=w270) -> (max value=w269:dbl)  [unwired: 3 out]
        n116 = case shown="False" w284 {
          tunnel: w283 -> [w295 _]
          tunnel: w282 -> [w294 w296]
          tunnel: [w293 w296] -> w281
          frame False {
            n117 = call-poly "Enqueue Message.vi"("error in (no error)"=w294, "Message"="Broadcast Settings", "Message Queue"=w295) -> ("error out"=w293:errorcluster)  [unwired: 7 in, 1 out]
          }
          frame True {
          }
        }
        n118 = call "Get Estimate Time.vi"("Speed"=w267, "Current SP"=0.0, "Next SP"=w269) -> ()  [unwired: 8 in, 1 out]
        n119 = call-poly "Name to ref convert.vi"("Array in"=string[] ["info"] ("name")) -> ("Array out"=w275:refnum<vi>[])  [unwired: 10 in]
        n120 = Index Array(array=w275) -> (element=w276:refnum<vi>)  [unwired: 1 in]
        n121 = Type Cast(type=refnum<vi> refnum ("LOG"), x=w276) -> (*(type *) &x=w279:refnum<vi>)
        n122 = disable-structure shown="Disabled" {
          disable-tunnel: w274 -> [w286 _]
          frame Disabled {
            n123 = call "Init Res Table.vi"() -> ()  [unwired: 12 in]
            n124 = call-poly "Name to ref convert.vi"("name"="RUN_Test") -> ("First REF"=w289:refnum<vi>)  [unwired: 10 in]
            n125 = Build Array(w289) -> (w288:refnum<vi>[])
            n126 = call "Set Enable State on Multiple Controls.vi"("Enable?"=w286, "Controls"=w288) -> ()  [unwired: 9 in, 1 out]
          }
          frame Enabled {
          }
        }
        n127 = disable-structure shown="Disabled" {
          disable-tunnel: w279 -> [w291 _]
          disable-tunnel: w277 -> [w290 _]
          frame Disabled {
            n128 = property class="Str"(reference=w291, "Value"=w290) -> ()  [unwired: 1 in, 2 out]
          }
          frame Enabled {
          }
        }
      }
      frame "Load Data File" {
        n129 = Variant To Data(type="*.tdms" ("format string"), Variant=w302) -> (data=w297:string)  [unwired: 1 in, 1 out]
        n130 = call "FGV Parameters.vi"("CMD"=PCT_FGV_CMD."GET", "Key"="Test File Name") -> ("output"=w300:variant)  [unwired: 7 in, 2 out]
        n131 = Variant To Data(type=path "Reports" ("name or relative path"), Variant=w300) -> (data=w298:path)  [unwired: 1 in, 1 out]
        n132 = disable-structure shown="Disabled" {
          disable-tunnel: w307 -> [w310 _]
          disable-tunnel: [w309 _] -> w306
          disable-tunnel: w298 -> [_ w341]
          disable-tunnel: w297 -> [_ w326]
          frame Disabled {
            n133 = disable-structure shown="Disabled" {
              disable-tunnel: [w321 _] -> w314
              disable-tunnel: w310 -> [w320 _]
              frame Disabled {
                n134 = call-poly <vilib>:"Set Cursor.vi"("error in (no error)"=w320, "icon"=u16 2) -> ("error out"=w321:errorcluster)  [unwired: 8 in, 1 out]
              }
              frame Enabled {
              }
            }
            n135 = call "File Dialog"("error in"=w314, "pattern (all files)"="*.tdms" ("format string")) -> ("selected path"=w315:path, "error out"=w313:errorcluster)  [unwired: 10 in, 2 out]
            n136 = call <vilib>:"Set Busy.vi"() -> ()  [unwired: 10 in, 2 out]
            n137 = call "Report Read RES Data File.vi"("error in (no error)"=w313, "RED Data File"=w315) -> ("error out"=w312:errorcluster)  [unwired: 9 in]
            n138 = disable-structure shown="Disabled" {
              disable-tunnel: w312 -> [w318 _]
              disable-tunnel: [w317 _] -> w311
              frame Disabled {
                n139 = call <vilib>:"Unset Busy.vi"("error in (no error)"=w318) -> ("error out"=w317:errorcluster)  [unwired: 10 in]
              }
              frame Enabled {
              }
            }
            n140 = call <vilib>:"Clear Errors.vi"("error in (no error)"=w311) -> ("error out"=w309:errorcluster)  [unwired: 5 in, 1 out]
          }
          frame Enabled {
            n141 = vi-ref "Data Dialog.vi"() -> (w332:refnum<vi>)
            n142 = property class="VI"(reference=w332) -> ("Name"=w336:string)  [unwired: 1 in, 2 out]
            n143 = Decimal String To Number(string=w326) -> (number=w322:i32)  [unwired: 2 in, 1 out]
            n144 = Open VI Reference(type specifier VI Refnum (for type only)=refnum<vi> refnum, vi path=w336, options=128 ("call and forget")) -> (vi reference=w335:refnum<vi>, error out=w330:errorcluster)  [unwired: 3 in]
            n145 = TDMS Open(6:FALSE ("disable buffering? (T)"), 10:T22."open (read-only)" ("operation"), 11:w341) -> (3:w340:refnum<k34>)  [unwired: 4 in, 1 out]
            n146 = TDMS Read(0:w340, 5:"Data" ("format string"), 12:dbl[][] [], 13:TRUE ("return channels in file order? (F)")) -> (8:w328:string[], 10:w325:dbl[][])  [unwired: 4 in, 4 out]
            n147 = Index Array(array=w325, index (row)=w322) -> (element=w324:dbl[])  [unwired: 1 in]
            n148 = Build Array(w324) -> (w323:dbl[][])
            n149 = call-by-ref "Start Asynchronous Call"(reference=w335, error in=w330, "channel name(s)"=w328, "Data"=w323) -> (reference out=w337:refnum<vi>, error out=w329:errorcluster)  [unwired: 9 in, 1 out]
            n150 = Close Reference(reference=w337, error in (no error)=w329) -> ()  [unwired: 1 out]
          }
        }
      }
      frame "Load PS Configuration" {
        # "Init UI Refs - Store control references for UI controls.  Also enable/disable controls appropriately."
        n151 = call "File Dialog2"("prompt"="Please select PS Configuration File", "default name"="PSConf.ini", "pattern (all files)"="*.ini") -> ("selected path"=w348:path, "cancelled"=w347:bool, "error out"=w343:errorcluster)  [unwired: 9 in, 1 out]
        n152 = case shown="False" w347 {
          tunnel: w348 -> [w352 _]
          tunnel: w343 -> [_ _]
          frame False {
            n153 = call "PalmSense Read Config File.vi"("configuration file path"=w352) -> ("error out"=w353:errorcluster)  [unwired: 10 in]
            n154 = call "DB Update Test Tree.vi"("error in (no error)"=w353) -> ()  [unwired: 10 in, 1 out]
          }
          frame True {
          }
        }
      }
      frame "LOG" {
        # "Start - Enable/Disable buttons appropriately for an acquisition that has started, and update status display."
        n155 = Variant To Data(type=TRUE, Variant=w360) -> (data=w355:bool)  [unwired: 1 in, 1 out]
        n156 = Select(t="Start" ("Message"), s=w355, f="Stop" ("Message")) -> (s? t:f=w357:string)
        n157 = call-poly "Enqueue Message.vi"("error in (no error)"=w364, "Message"=w357, "Message Queue"=w362) -> ("error out"=w361:errorcluster)  [unwired: 7 in, 1 out]
      }
      frame "Logging Stopped" {
        # "Logic for determining what action to take when the logging has stopped."
      }
      frame "Main Menu Value Change" {
        # "Broadcast settings - Send the 'Update Settings' message to the Logging and Acquisition message loops."
        n158 = Variant To Data(type=Main_Menu_Selector."Main Screen" ("Main Menu"), Variant=w372) -> (data=w369:T23)  [unwired: 1 in, 1 out]
        n159 = case shown="\"Test Setting\"" w369 {
          tunnel: w368 -> [w376 w380 w383]
          frame "Main Screen", Default {
            n160 = call-poly "Enqueue Message.vi"("Message Data"=enum32{"Test", "History"}."Test" ("Switch Main Tab"), "Message"="Main Tab Switch", "Message Queue"=w376) -> ()  [unwired: 7 in, 2 out]
          }
          frame "Test Setting" {
            n161 = call-poly "Enqueue Message.vi"("Message"="Launch Settings Dialog", "Message Queue"=w380) -> ()  [unwired: 8 in, 2 out]
          }
          frame "History" {
            n162 = call-poly "Enqueue Message.vi"("Message Data"=enum32{"Test", "History"}."History" ("Switch Main Tab"), "Message"="Main Tab Switch", "Message Queue"=w383) -> ()  [unwired: 7 in, 2 out]
          }
        }
        n163 = Merge Errors(w374) -> (w375:errorcluster)
      }
      frame "Main Tab Switch" {
        # "Start - Enable/Disable buttons appropriately for an acquisition that has started, and update status display."
        n164 = Variant To Data(type=enum32{"Test", "History"}."Test" ("Switch Main Tab"), Variant=w389) -> (data=w384:enum32{"Test", "History"})  [unwired: 1 in, 1 out]
        n165 = call-poly "Name to ref convert.vi"("Array in"=string[] ["Display Tab"] ("name")) -> ("Array out"=w396:refnum<vi>[])  [unwired: 10 in]
        n166 = Index Array(array=w396) -> (element #1=w392:refnum<vi>)  [unwired: 2 in, 1 out]
        n167 = call "PCT Configure Enqueue CMD.vi"("Parameter Data"=w389, "CMD"=T4 {"Type CMD"="Mode", "Mode CMD"="", "Main CMD"="Action-Status"}, "CMD Queue in"=w390) -> ()  [unwired: 6 in, 3 out]
        n168 = To More Specific Class(target class=refnum<vi> refnum ("Display Tab"), reference=w392) -> (specific class reference=w393:refnum<vi>)  [unwired: 1 in, 1 out]
        n169 = case shown="\"History\"" w384 {
          tunnel: w385 -> [_ w399]
          frame "Test", Default {
          }
          frame "History" {
            n170 = call-poly "Enqueue Message.vi"("Message"="DB Get Tests Details" ("name"), "Message Queue"=w399) -> ()  [unwired: 8 in, 2 out]
          }
        }
        n171 = property class="TabCtl (strict)"(reference=w393, "Value"=w384) -> ()  [unwired: 1 in, 2 out]
      }
      frame "Manual Channel Switch" {
        (unwired) T32."1" ("NewVal")
        # "Start - Enable/Disable buttons appropriately for an acquisition that has started, and update status display."
        n172 = Variant To Data(type=T24 {"Back-Front Switch"=FALSE, "NewVal"=enum."1"} ("output cluster"), Variant=w417) -> (data=w411:T24)  [unwired: 1 in, 1 out]
        n173 = Unbundle(w411) -> ("Back-Front Switch"=w403:bool, "NewVal"=w404:T32)
        n174 = Increment(x=w404) -> (x+1=w409:T32)
        n175 = Unbundle By Name(w416) -> ("Answer"=w413:refnum<queue>, "PalmSens"=w415:refnum<queue>)
        n176 = Add(x=w409, y=100) -> (x+y=w408:u32)
        n177 = Number To Decimal String(number=w408) -> (decimal integer string=w406:string)  [unwired: 1 in]
        n178 = Flush Queue(queue=w413) -> (queue out=w401:refnum<queue>)  [unwired: 1 in, 2 out]
        n179 = Bundle By Name(cluster=cluster{"Channel":string, "Backplane":bool} {"Channel"="101:106", "Backplane"=FALSE}, "Backplane"=w403, "Channel"=w406) -> (w402:cluster{"Channel":string, "Backplane":bool})
        n180 = call "PCT Configure Enqueue CMD.vi"("Response Queue"=w401, "Parameter Data"=w402, "Read"=FALSE, "CMD"=T4 {"Type CMD"="Switch", "Mode CMD"="", "Main CMD"="Action-Status"}, "CMD Queue in"=w415) -> ()  [unwired: 4 in, 3 out]
      }
      frame "Manual GO POS" {
        # "Start - Enable/Disable buttons appropriately for an acquisition that has started, and update status display."
        n181 = Unbundle By Name(w429) -> ("XYZ notifier"=w428:refnum<notifier>)
        n182 = call <vilib>:"Set Busy.vi"("VI reference (current VI)"=w421) -> ("error out"=w423:errorcluster)  [unwired: 9 in, 1 out]
        n183 = call "Send Go  POS.vi"("Type CMD"="GoToPos All", "Parameter Data"=w427, "XYZ notifier"=w428, "error in (no error)"=w423, "Motor Queue in"=w436) -> ("error out"=w422:errorcluster)  [unwired: 5 in, 1 out]
        n184 = Variant To Data(type=cluster{"dX":dbl, "dY":dbl, "dZ":dbl, "dA":dbl} {"dX"=150.0, "dY"=150.0, "dZ"=150.0, "dA"=150.0} ("Set Position"), Variant=w427) -> (data=w425:cluster{"dX":dbl, "dY":dbl, "dZ":dbl, "dA":dbl})  [unwired: 1 in, 1 out]
        n185 = disable-structure shown="Disabled" {
          disable-tunnel: w434 -> [w438 _]
          frame Disabled {
            n186 = Unbundle By Name(w438) -> ("OPC"=w439:refnum<queue>)
            n187 = call "Check OPC.vi"("OPC Queue"=w439) -> ()  [unwired: 10 in, 1 out]
          }
          frame Enabled {
          }
        }
        n188 = Cluster To Array(cluster=w425) -> (array=w424:dbl[])
        n189 = call <vilib>:"Unset Busy.vi"("error in (no error)"=w422, "VI reference (current VI)"=w421) -> ()  [unwired: 9 in, 1 out]
        n190 = call "Bundle CMD Queue Cluster.vi"("Message Data"=w424, "Message"="Update XY Graph" ("Type CMD")) -> ("Message Cluster"=w433:T29)  [unwired: 9 in]
        n191 = call-poly "Enqueue Message.vi"("Message Data"=w433, "Message"="Update Status" ("Main CMD"), "Message Queue"=w430) -> ()  [unwired: 7 in, 2 out]
      }
      frame "Manual MFC Select Gas" {
        # "Start - Enable/Disable buttons appropriately for an acquisition that has started, and update status display."
        n192 = Variant To Data(type="SetPoint" ("Type CMD"), Variant=w442) -> ()  [unwired: 1 in, 2 out]
        n193 = Unbundle By Name(w441) -> ("MFC"=w440:refnum<queue>)
        n194 = call "PCT Configure Enqueue CMD.vi"("Parameter Data"=w442, "CMD"=T4 {"Type CMD"="Select gas", "Mode CMD"="Gas", "Main CMD"="Configure"}, "CMD Queue in"=w440) -> ()  [unwired: 6 in, 3 out]
      }
      frame "Manual MFC Setpoint" {
        (unwired) refnum<vi> refnum ("element")
        # "Start - Enable/Disable buttons appropriately for an acquisition that has started, and update status display."
        n195 = Variant To Data(type=refnum<vi> refnum ("Set Point Options"), Variant=w454) -> (data=w451:refnum<vi>)  [unwired: 1 in, 1 out]
        n196 = property class="Clust (strict)"(reference=w451) -> ("Controls[]"=w450:refnum<vi>[])  [unwired: 1 in, 2 out]
        n197 = Unbundle By Name(w449) -> ("MFC"=w448:refnum<queue>)
        n198 = for {
          tunnel: w448 -> [w462]
          tunnel: w450 -> [w457] mode=indexing
          n199 = property class="Ctl"(reference=w457) -> ("Label.Text"=w458:string, "Value"=w460:variant)  [unwired: 1 in, 2 out]
          n200 = Bundle By Name(cluster=T4 {"Type CMD"="SetPoint", "Mode CMD"="", "Main CMD"="Configure"} ("CMD"), "Mode CMD"=w458) -> (w459:T4)
          n201 = call "PCT Configure Enqueue CMD.vi"("Parameter Data"=w460, "CMD"=w459, "CMD Queue in"=w462) -> ()  [unwired: 6 in, 3 out]
        }
      }
      frame "Manual Motor Stop" {
        # "Start - Enable/Disable buttons appropriately for an acquisition that has started, and update status display."
        n202 = disable-structure shown="Enabled" {
          disable-tunnel: w466 -> [w477 _]
          disable-tunnel: w464 -> [w473 w478]
          disable-tunnel: w463 -> [w470 _]
          frame Disabled {
            n203 = Variant To Data(type=i16 0 ("SET POS"), Variant=w477) -> ()  [unwired: 1 in, 2 out]
            n204 = call "PCT Configure Enqueue CMD.vi"("CMD"=T4 {"Type CMD"="Reset", "Mode CMD"="Counter", "Main CMD"="Utility"}, "CMD Queue in"=w473) -> ("CMD Queue out"=w472:refnum<queue>)  [unwired: 7 in, 2 out]
            n205 = call "PCT Configure Enqueue CMD.vi"("CMD"=T4 {"Type CMD"="Reset", "Mode CMD"="General", "Main CMD"="Utility"}, "CMD Queue in"=w472) -> ("error out"=w469:errorcluster)  [unwired: 7 in, 2 out]
            n206 = Unbundle By Name(w470) -> ("OPC"=w471:refnum<queue>)
            n207 = call "Check OPC.vi"("error in (no error)"=w469, "OPC Queue"=w471) -> ()  [unwired: 9 in, 1 out]
          }
          frame Enabled {
            n208 = call "PCT Configure Enqueue CMD.vi"("Parameter Data"=0.0 ("y"), "CMD"=T4 {"Type CMD"="Program Stop", "Mode CMD"="", "Main CMD"="Action-Status"}, "CMD Queue in"=w478) -> ()  [unwired: 6 in, 3 out]
          }
        }
      }
      frame "Manual PS Scan" {
        # "Start - Enable/Disable buttons appropriately for an acquisition that has started, and update status display."
        n209 = Unbundle By Name(w493) -> ("PS Data Queue"=w492:refnum<queue>, "PLC AI Notifier"=w491:refnum<notifier>, "PLC DI notifier"=w490:refnum<notifier>)
        n210 = Unbundle By Name(w484) -> ("PalmSense  Configuration.Method.Name"=w482:string)
        n211 = Send Notification(notification=bool[] [TRUE], notifier=w490) -> (notifier out=w485:refnum<notifier>, error out=w487:errorcluster)  [unwired: 1 in]
        n212 = call "PS long Name to Short.vi"("String"=w482) -> ("whole match"=w481:string)  [unwired: 10 in]
        n213 = call "Scope Get Trace State Machine.vi"("Type Measurement"=w481, "error in (no error)"=w487, "Data Queue"=w492, "Queue in"=w494) -> ("error out"=w483:errorcluster, "Measurements"=w489:dbl[])  [unwired: 5 in, 1 out]
        n214 = Send Notification(notification=bool[] [FALSE], notifier=w485, error in (no error)=w483) -> ()  [unwired: 2 out]
        n215 = disable-structure shown="Disabled" {
          disable-tunnel: w483 -> [w499 _]
          frame Disabled {
            n216 = call-poly "Name to ref convert.vi"("name"="PS Scan") -> ("First REF"=w501:refnum<vi>)  [unwired: 10 in]
            n217 = To More Specific Class(target class=refnum<vi> refnum ("PS Scan"), reference=w501) -> (specific class reference=w498:refnum<vi>)  [unwired: 1 in, 1 out]
            n218 = property class="Bool (strict)"(reference=w498, error in=w499, "Value"=FALSE ("Visible")) -> ()  [unwired: 2 out]
          }
          frame Enabled {
          }
        }
        n219 = Send Notification(notification=w489, notifier=w491) -> ()  [unwired: 1 in, 2 out]
      }
      frame "Manual SET POS" {
        # "Start - Enable/Disable buttons appropriately for an acquisition that has started, and update status display."
        n220 = Variant To Data(type=i16 0 ("SET POS"), Variant=w508) -> (data=w504:i16)  [unwired: 1 in, 1 out]
        n221 = call "PCT Configure Enqueue CMD.vi"("Parameter Data"=w504, "CMD"=T4 {"Type CMD"="Position", "Mode CMD"="", "Main CMD"="Configure"}, "CMD Queue in"=w506) -> ()  [unwired: 6 in, 3 out]
      }
      frame "Manual SET Reset" {
        # "Start - Enable/Disable buttons appropriately for an acquisition that has started, and update status display."
        n222 = call <vilib>:"Set Busy.vi"("VI reference (current VI)"=w514) -> ("error out"=w515:errorcluster)  [unwired: 9 in, 1 out]
        n223 = call-poly "Name to ref convert.vi"("name"="PLC Reset") -> ("First REF"=w522:refnum<vi>)  [unwired: 10 in]
        n224 = Unbundle By Name(w544) -> ("XYZ notifier"=w533:refnum<notifier>)
        n225 = Build Array(w522) -> (w519:refnum<vi>[])
        n226 = call-poly "Name to ref convert.vi"("name"="Set Position") -> ("First REF"=w531:refnum<vi>)  [unwired: 10 in]
        n227 = Array To Cluster(array=i32[] []) -> (cluster=w543:cluster{"[0]":i32, "[1]":i32})
        n228 = call-poly "Name to ref convert.vi"("name"="XY Graph") -> ("First REF"=w537:refnum<vi>)  [unwired: 10 in]
        n229 = call "Set Enable State on Multiple Controls.vi"("Enable?"=FALSE, "Controls"=w519) -> ("error out"=w520:errorcluster)  [unwired: 9 in]
        n230 = Unbundle(w543) -> ("[0]"=w542:i32, "[1]"=w541:i32)
        n231 = To More Specific Class(target class=refnum<vi> refnum ("Set Position"), reference=w531) -> (specific class reference=w529:refnum<vi>)  [unwired: 1 in, 1 out]
        n232 = To More Specific Class(target class=refnum<vi> refnum ("XY Graph"), reference=w537) -> (specific class reference=w536:refnum<vi>)  [unwired: 1 in, 1 out]
        n233 = Merge Errors(w515, w520) -> (w516:errorcluster)
        n234 = call "Build XY Graph3"("Reset"=FALSE, "Y Input"=w541, "X Input"=w542) -> ("XY Graph"=w540:cluster{"X":dbl[], "Y":dbl[]}[])  [unwired: 7 in, 1 out]
        n235 = property class="Clust (strict)"(reference=w529) -> ("Controls[]"=w528:refnum<vi>[])  [unwired: 1 in, 2 out]
        n236 = call "Tango Reset.vi"("error in (no error)"=w516, "XYZ notifier"=w533, "Queue in"=w511) -> ("error out"=w513:errorcluster, "Measurements"=w527:dbl[])  [unwired: 6 in, 1 out]
        n237 = property class="XYGraph (strict)"(reference=w536, "Value"=w540) -> ()  [unwired: 1 in, 2 out]
        n238 = call "Send to Home.vi"("error in (no error)"=w513, "Mototr Queue in"=w511) -> ("error out"=w512:errorcluster)  [unwired: 8 in, 1 out]
        n239 = call "Set Enable State on Multiple Controls.vi"("error in (no error)"=w512, "Enable?"=TRUE, "Controls"=w519) -> ()  [unwired: 8 in, 1 out]
        n240 = disable-structure shown="Enabled" {
          disable-tunnel: w527 -> [w550 w551]
          disable-tunnel: [w549 w551] -> w517
          frame Disabled {
            n241 = Divide(x=w550, y=2.0 ("Numeric")) -> (x/y=w549:dbl[])
          }
          frame Enabled {
          }
        }
        n242 = Build Array (concatenate)(w527, 50.0 ("Numeric")) -> (w525:dbl[])
        n243 = for {
          tunnel: w528 -> [w556] mode=indexing
          tunnel: w525 -> [w553] mode=indexing
          tunnel: dbl[] [0.0, 0.0, -50.0] -> [w552] mode=indexing
          n244 = To More Specific Class(target class=refnum<vi> refnum ("dX"), reference=w556) -> (specific class reference=w555:refnum<vi>)  [unwired: 1 in, 1 out]
          n245 = property class="DigNum (strict)"(reference=w555, "Maximum"=w553, "Minimum"=w552) -> ()  [unwired: 1 in, 2 out]
        }
        n246 = for {
          tunnel: w517 -> [w557] mode=indexing
          i -> [w558]
          n247 = call "FGV GAGE Zero.vi"("CMD"=PCT_FGV_CMD."SET", "index"=w558, "input"=w557) -> ()  [unwired: 7 in, 2 out]
        }
        n248 = call <vilib>:"Unset Busy.vi"("error in (no error)"=w512, "VI reference (current VI)"=w514) -> ()  [unwired: 9 in, 1 out]
      }
      frame "Manual SET VEL" {
        # "Start - Enable/Disable buttons appropriately for an acquisition that has started, and update status display."
        n249 = Variant To Data(type=0.0 ("SET POS"), Variant=w564) -> (data=w561:dbl)  [unwired: 1 in, 1 out]
        n250 = Bundle By Name(cluster=cluster{"dX":dbl, "dY":dbl, "dZ":dbl, "dA":dbl} {"dX"=0.0, "dY"=0.0, "dZ"=0.0, "dA"=0.0} ("input cluster"), "dX"=w561, "dY"=w561, "dZ"=w561, "dA"=w561) -> (w560:cluster{"dX":dbl, "dY":dbl, "dZ":dbl, "dA":dbl})
        n251 = call "PCT Configure Enqueue CMD.vi"("Parameter Data"=w560, "CMD"=T4 {"Type CMD"="Speed", "Mode CMD"="", "Main CMD"="Configure"}, "CMD Queue in"=w566) -> ()  [unwired: 6 in, 3 out]
      }
      frame "Manual Start Motor" {
        # "Start - Enable/Disable buttons appropriately for an acquisition that has started, and update status display."
        n252 = call "PCT Configure Enqueue CMD.vi"("Parameter Data"=w573, "CMD"=T4 {"Type CMD"="Start", "Mode CMD"="", "Main CMD"="Action-Status"}, "CMD Queue in"=w572) -> ()  [unwired: 6 in, 3 out]
      }
      frame "Manual Start Scan" {
        # "Start - Enable/Disable buttons appropriately for an acquisition that has started, and update status display."
        n253 = Unbundle By Name(w578) -> ("HIDEN"=w576:refnum<queue>)
        n254 = Variant To Data(type=TRUE, Variant=w581) -> (data=w577:bool)  [unwired: 1 in, 1 out]
        n255 = case shown="True" w577 {
          tunnel: w576 -> [w586 w592]
          frame False {
            n256 = call "PCT Configure Enqueue CMD.vi"("Parameter Data"=0, "CMD"=T4 {"Type CMD"="Stop Scan", "Mode CMD"="", "Main CMD"="Action-Status"}, "CMD Queue in"=w586) -> ()  [unwired: 6 in, 3 out]
          }
          frame True {
            n257 = call "Update Hiden Scan Details.vi"("Queue in"=w592) -> ("Queue Out"=w590:refnum<queue>)  [unwired: 10 in]
            n258 = call "PCT Configure Enqueue CMD.vi"("Parameter Data"=0, "CMD"=T4 {"Type CMD"="Start Scan", "Mode CMD"="", "Main CMD"="Action-Status"}, "CMD Queue in"=w590) -> ("CMD Queue out"=w587:refnum<queue>)  [unwired: 6 in, 2 out]
            n259 = call "PCT Configure Enqueue CMD.vi"("CMD"=T4 {"Type CMD"="", "Mode CMD"="", "Main CMD"="Data"}, "CMD Queue in"=w587) -> ()  [unwired: 7 in, 3 out]
          }
        }
      }
      frame "Manual Valve Pressed" {
        w593 = "Start" ("name")
        # "Start - Enable/Disable buttons appropriately for an acquisition that has started, and update status display."
        n260 = Variant To Data(type=T25 {"Writer Queue"=refnum, "Timeout"=[], "Status"=[]}, Variant=w604) -> (data=w597:T25)  [unwired: 1 in, 1 out]
        n261 = Unbundle By Name(w597) -> ("Status"=w596:bool[])
        n262 = Bundle By Name(cluster=w597, "Writer Queue"=w602) -> (w601:T25)
        n263 = Unbundle By Name(w600) -> ("VALVE"=w599:refnum<queue>)
        n264 = Or Array Elements(Boolean array=w596) -> (logical OR=w595:bool)
        n265 = Select(t=w593, s=w595, f="Stop" ("name")) -> ()  [unwired: 1 out]
        n266 = call-poly "Enqueue Message.vi"("Message Data"=w601, "Message"=w593, "Message Queue"=w599) -> ()  [unwired: 7 in, 2 out]
      }
      frame "Manual XYZ Configure" {
        # "Start - Enable/Disable buttons appropriately for an acquisition that has started, and update status display."
        n267 = call "PCT Configure Enqueue CMD.vi"("Parameter Data"="Absolute" ("Position Mode"), "CMD"=T4 {"Type CMD"="Position Mode", "Mode CMD"="", "Main CMD"="Configure"}, "CMD Queue in"=w609) -> ()  [unwired: 6 in, 3 out]
      }
      frame "Pause Process" {
        # "Start - Enable/Disable buttons appropriately for an acquisition that has started, and update status display."
        n268 = call-poly "Name to ref convert.vi"("name"="Stop Process") -> ("First REF"=w614:refnum<vi>)  [unwired: 10 in]
        n269 = property class="Ctl"(reference=w614, "Visible"=TRUE) -> ()  [unwired: 1 in, 2 out]
        n270 = call-poly "Enqueue Message.vi"("Priority Message? (F)"=TRUE, "Message"="Procedure Pause", "Message Queue"=w620) -> ("error out"=w621:errorcluster)  [unwired: 7 in, 1 out]
      }
      frame "PLC Reset Error" {
        # "Start - Enable/Disable buttons appropriately for an acquisition that has started, and update status display."
        n271 = Variant To Data(type=TRUE, Variant=w633) -> ()  [unwired: 1 in, 2 out]
        n272 = disable-structure shown="Disabled" {
          frame Disabled {
            n273 = call-poly "Name to ref convert.vi"("name"="Reset Error") -> ("First REF"=w636:refnum<vi>)  [unwired: 10 in]
            n274 = property class="Ctl"(reference=w636, "Visible"=FALSE) -> ()  [unwired: 1 in, 2 out]
          }
          frame Enabled {
          }
        }
        n275 = Bundle By Name(cluster=T27 {"Channels"=enum."Polling_Cylinder", "Status"=FALSE}, "Channels"=T26."Reset_Error" ("Enum"), "Status"=TRUE) -> (w626:T27)
        n276 = call-poly "Enqueue Message.vi"("error in (no error)"=w630, "Message Data"=w626, "Message"="Write Coil", "Message Queue"=w623) -> ("error out"=w629:errorcluster)  [unwired: 6 in, 1 out]
      }
      frame "Popup Keyboard" {
        (unwired) refnum<vi> refnum  # Ctrl REF
        n277 = Variant To Data(type=refnum<vi> refnum ("Digital in REF"), Variant=w651) -> (data=w648:refnum<vi>)  [unwired: 1 in, 1 out]
        n278 = Unbundle By Name(w647) -> ("Answer"=w646:refnum<queue>)
        n279 = property class="Num"(reference=w648) -> (reference out=w649:refnum<vi>, "Label.Text"=w650:string, "Maximum"=w639:dbl, "Minimum"=w638:dbl)  [unwired: 1 in, 1 out]
        n280 = call "KB numeric.vi"("Parameters name"=w650) -> ("cancel?"=w645:bool, "password"=w652:string)  [unwired: 9 in]
        n281 = Fract/Exp String To Number(string=w652) -> (number=w641:dbl)  [unwired: 3 in, 1 out]
        n282 = In Range and Coerce(upper limit=w639, x=w641, lower limit=w638) -> (coerced(x)=w640:dbl)  [unwired: 1 out]
        n283 = case shown="True" w645 {
          tunnel: w649 -> [w656 _]
          tunnel: w640 -> [w655 _]
          frame False {
            n284 = property class="Num"(reference=w656, "Value"=w655) -> ()  [unwired: 1 in, 2 out]
          }
          frame True {
          }
        }
        n285 = Bundle("Maximum"=w640, "cancel?"=w645) -> (w644:cluster{"Maximum":dbl, "cancel?":bool})  [unwired: 1 in]
        n286 = call-poly "Enqueue Message.vi"("Message Data"=w644, "Message"=w643, "Message Queue"=w646) -> ()  [unwired: 7 in, 2 out]
      }
      frame "Position Mode" {
        # "Start - Enable/Disable buttons appropriately for an acquisition that has started, and update status display."
        n287 = call "PCT Configure Enqueue CMD.vi"("Parameter Data"=w658, "CMD"=T4 {"Type CMD"="Position Mode", "Mode CMD"="", "Main CMD"="Configure"}, "CMD Queue in"=w660) -> ()  [unwired: 6 in, 3 out]
      }
      frame "Pump Set Speed" {
        # "Start - Enable/Disable buttons appropriately for an acquisition that has started, and update status display."
        n288 = call "PCT Configure Enqueue CMD.vi"("Parameter Data"=w665, "CMD"=T4 {"Type CMD"="Speed", "Mode CMD"="", "Main CMD"="Configure"}, "CMD Queue in"=w666) -> ()  [unwired: 6 in, 3 out]
      }
      frame "Pump Reverse Direction" {
        # "Start - Enable/Disable buttons appropriately for an acquisition that has started, and update status display."
        n289 = call "PCT Configure Enqueue CMD.vi"("Parameter Data"=w671, "CMD"=T4 {"Type CMD"="Reverse Direction", "Mode CMD"="", "Main CMD"="Action-Status"}, "CMD Queue in"=w672) -> ()  [unwired: 6 in, 3 out]
      }
      frame "Pump Start" {
        # "Start - Enable/Disable buttons appropriately for an acquisition that has started, and update status display."
        n290 = call "PCT Configure Enqueue CMD.vi"("Parameter Data"=w677, "CMD"=T4 {"Type CMD"="Run", "Mode CMD"="", "Main CMD"="Action-Status"}, "CMD Queue in"=w678) -> ()  [unwired: 6 in, 3 out]
      }
      frame "Pump Set Direction" {
        w689 = u16 1 items=["CW", "CCW"] ("Direction")
        w688 = u16 0 items=["CW", "CCW"] ("Direction")
        # "Start - Enable/Disable buttons appropriately for an acquisition that has started, and update status display."
        n291 = Variant To Data(type="", Variant=w683) -> (data=w685:string)  [unwired: 1 in, 1 out]
        n292 = Equal?(x=w685, y="CW") -> (x = y?=w687:bool)
        n293 = Select(t=w688, s=w687, f=w689) -> (s? t:f=w682:u16)
        n294 = call "PCT Configure Enqueue CMD.vi"("Parameter Data"=w682, "CMD"=T4 {"Type CMD"="Direction", "Mode CMD"="", "Main CMD"="Configure"}, "CMD Queue in"=w691) -> ()  [unwired: 6 in, 3 out]
      }
      frame "Pump Change Speed" {
        # "Start - Enable/Disable buttons appropriately for an acquisition that has started, and update status display."
        n295 = Variant To Data(type="", Variant=w695) -> (data=w698:string)  [unwired: 1 in, 1 out]
        n296 = Bundle By Name(cluster=T4 {"Type CMD"="Change Speed", "Mode CMD"="", "Main CMD"="Action-Status"} ("CMD"), "Mode CMD"=w698) -> (w694:T4)
        n297 = call "PCT Configure Enqueue CMD.vi"("Parameter Data"=w695, "CMD"=w694, "CMD Queue in"=w700) -> ()  [unwired: 6 in, 3 out]
      }
      frame "Pump Get Info" {
        # "Start - Enable/Disable buttons appropriately for an acquisition that has started, and update status display."
        n298 = call-poly "Name to ref convert.vi"("name"="Pump Info") -> ("First REF"=w703:refnum<vi>)  [unwired: 10 in]
        n299 = To More Specific Class(target class=refnum<vi> refnum ("Pump Info"), reference=w703) -> (specific class reference=w713:refnum<vi>)  [unwired: 1 in, 1 out]
        n300 = call "Obtain Message Queue.vi"() -> ("Message Queue"=w705:refnum<queue>)  [unwired: 10 in, 1 out]
        n301 = property class="Clust (strict)"(reference=w713) -> (reference out=w714:refnum<vi>, "Value"=w711:T33)  [unwired: 1 in, 1 out]
        n302 = call "PCT Configure Enqueue CMD.vi"("Response Queue"=w705, "Parameter Data"=w716, "Read"=TRUE, "CMD"=T4 {"Type CMD"="", "Mode CMD"="Info", "Main CMD"="Data"}, "CMD Queue in"=w717) -> ("error out"=w707:errorcluster, "Message Data"=w710:variant)  [unwired: 4 in, 1 out]
        n303 = Release Queue(queue=w705, error in (no error)=w707) -> ()  [unwired: 1 in, 3 out]
        n304 = Variant To Data(type=w711, Variant=w710) -> (data=w709:T33)  [unwired: 1 in, 1 out]
        n305 = property class="Clust (strict)"(reference=w714, "Value"=w709) -> ()  [unwired: 1 in, 2 out]
      }
      frame "PS Measure Type Update" {
        # "Init UI Refs - Store control references for UI controls.  Also enable/disable controls appropriately."
        n306 = Variant To Data(type="", Variant=w734) -> (data=w722:string)  [unwired: 1 in, 1 out]
        n307 = call-poly "Name to ref convert.vi"("name"="PS Measure Type") -> ("First REF"=w735:refnum<vi>)  [unwired: 10 in]
        n308 = To More Specific Class(target class=refnum<vi> refnum ("PS Measure Type 2"), reference=w735) -> (specific class reference=w732:refnum<vi>)  [unwired: 1 in, 1 out]
        n309 = call-poly "Name to ref convert.vi"("name"="PS Measure Type List") -> ("First REF"=w727:refnum<vi>)  [unwired: 10 in]
        n310 = call "PS Get MEasure Params.vi"("Ring Text"=w722, "PS Measure Type 2"=w732) -> ()  [unwired: 10 in]
        n311 = To More Specific Class(target class=refnum<vi> refnum ("PS Measure Type List"), reference=w727) -> (specific class reference=w724:refnum<vi>)  [unwired: 1 in, 1 out]
        n312 = property class="Ring (strict)"(reference=w724) -> (reference out=w721:refnum<vi>, "Strings []"=w723:string[])  [unwired: 1 in, 1 out]
        n313 = call "FGV Parameters.vi"("CMD"=PCT_FGV_CMD."SET", "input"=w722, "Key"="PS Name Scan") -> ()  [unwired: 6 in, 3 out]
        n314 = Bundle By Name(cluster=w739, "PalmSense  Configuration.Method.Name"=w722) -> (w731:T7)
        n315 = Search 1D Array(1D array=w723, element=w722) -> (index of element=w720:i32)  [unwired: 1 in]
        n316 = property class="Ring (strict)"(reference=w721, "Value"=w720) -> ()  [unwired: 1 in, 2 out]
      }
      frame "PS Save Measurements" {
        # "Start - Enable/Disable buttons appropriately for an acquisition that has started, and update status display."
      }
      frame "PS Scan Update" {
        # "Init UI Refs - Store control references for UI controls.  Also enable/disable controls appropriately."
        n317 = call "PalmSense Save Config File.vi"() -> ()  [unwired: 11 in, 1 out]
      }
      frame "Report  Send" {
        # "Broadcast settings - Send the 'Update Settings' message to the Logging and Acquisition message loops."
        n318 = Variant To Data(type=cluster{bool, "Data File Path":path} {TRUE, "Data File Path"=path ""}, Variant=w751) -> (data=w749:cluster{bool, "Data File Path":path})  [unwired: 1 in, 1 out]
        n319 = Unbundle(w749) -> (w748:bool, "Data File Path"=w747:path)
        n320 = Unbundle By Name(w757) -> ("Report Configuration"=w753:T15)
        n321 = Unbundle By Name(w755) -> ("Report"=w754:refnum<queue>)
        n322 = Bundle By Name(cluster=w753, "Popup Dialog"=w748, "Data File Path"=w747) -> (w752:T15)
        n323 = call-poly "Enqueue Message.vi"("Message Data"=w752, "Message"="Start", "Message Queue"=w754) -> ()  [unwired: 7 in, 2 out]
        n324 = Merge Errors(w758) -> (w759:errorcluster)
      }
      frame "Send PLC Home" {
        n325 = call <vilib>:"Set Busy.vi"("VI reference (current VI)"=w762) -> ("error out"=w764:errorcluster)  [unwired: 9 in, 1 out]
        n326 = call "Send to Home.vi"("error in (no error)"=w764, "Mototr Queue in"=w767) -> ("error out"=w763:errorcluster, "Mototr Queue out"=w760:refnum<queue>)  [unwired: 8 in]
        n327 = call <vilib>:"Unset Busy.vi"("error in (no error)"=w763, "VI reference (current VI)"=w762) -> ()  [unwired: 9 in, 1 out]
        n328 = disable-structure shown="Disabled" {
          disable-tunnel: w765 -> [w772 _]
          disable-tunnel: w763 -> [w770 _]
          frame Disabled {
            n329 = Unbundle By Name(w772) -> ("OPC"=w771:refnum<queue>)
            n330 = call "Check OPC.vi"("error in (no error)"=w770, "OPC Queue"=w771) -> ()  [unwired: 9 in, 1 out]
          }
          frame Enabled {
          }
        }
        n331 = call "PCT Configure Enqueue CMD.vi"("CMD"=T4 {"Type CMD"="GetPos", "Mode CMD"="GetPos", "Main CMD"="Data"}, "CMD Queue in"=w760) -> ()  [unwired: 7 in, 3 out]
      }
      frame "Sign In" {
        w773 = string[] ["1", "2", "1", "Eugene"] ("User Data")
        n332 = disable-structure shown="Default" {
          disable-tunnel: [w785 w790] -> _
          disable-tunnel: w778 -> [_ w789]
          disable-tunnel: [errorcluster {"status"=FALSE, "code"=0, "source"=""} ("error out") w788] -> w780
          disable-tunnel: string[] ["1", "2", "1", "Eugene"] ("User Data") -> [w785 w787]
          frame condition #0 (active) {
          }
          frame condition #1 {
            n333 = disable-structure shown="Enabled" {
              disable-tunnel: [w793 w794] -> w790
              disable-tunnel: w789 -> [w792 _]
              disable-tunnel: [w791 _] -> w788
              disable-tunnel: w787 -> [_ w794]
              frame Disabled {
                n334 = call "Get User and Password Event.vi"("Error In"=w792) -> ("Error Out"=w791:errorcluster, "User Data"=w793:string[])  [unwired: 8 in, 1 out]
              }
              frame Enabled {
              }
            }
          }
        }
        n335 = Index Array(array=w773, index=3) -> (element=w776:string)
        n336 = call-poly "Enqueue Message.vi"("error in (no error)"=w778, "Message Data"=w780, "Message"="Check Authorization", "Message Queue"=w782) -> ("error out"=w779:errorcluster)  [unwired: 6 in, 1 out]
        n337 = Bundle By Name(cluster=w784, "Support.User Details"=w773, "Process.Test Configuration.System Preset.Test Configuration.Operator"=w776) -> (w783:T7)
      }
      frame "Start Process" {
        # "Start - Enable/Disable buttons appropriately for an acquisition that has started, and update status display."
        n338 = case shown="\"Idle\", Default" w797 {
          tunnel: [w808 w838] -> w801
          tunnel: w800 -> [w807 w835]
          tunnel: w799 -> [w806 w838]
          tunnel: w798 -> [w804 _]
          tunnel: w796 -> [w803 _]
          tunnel: w795 -> [w802 _]
          frame "Idle", Default {
            n339 = call "Prepare Version Info.vi"("Settings"=w804) -> ("Enable"=w805:bool)  [unwired: 7 in, 3 out]
            n340 = case shown="True" w805 {
              tunnel: [w812 w829] -> w808
              tunnel: w807 -> [_ w828]
              tunnel: w806 -> [w812 w826]
              tunnel: w804 -> [_ w819]
              tunnel: w803 -> [_ w818]
              tunnel: w802 -> [_ _]
              frame False {
                n341 = call "Display Message to User"() -> ()  [unwired: 10 in, 2 out]
                n342 = call-poly "Name to ref convert.vi"("name"="Start Process") -> ("First REF"=w810:refnum<vi>)  [unwired: 10 in]
                n343 = property class="Ctl"(reference=w810, "Value"=FALSE ("Visible")) -> ()  [unwired: 1 in, 2 out]
              }
              frame True {
                (unwired) Test_Type."Test" ("Test Type")
                n344 = Unbundle By Name(w819) -> ("Process.Test Configuration.Test Type"=w817:T14)
                n345 = disable-structure shown="Disabled" {
                  disable-tunnel: w818 -> [w831 _]
                  frame Disabled {
                    n346 = call "PCT Configure Enqueue CMD.vi"("CMD"=T4 {"Type CMD"="Reset", "Mode CMD"="Counter", "Main CMD"="Utility"}, "CMD Queue in"=w831) -> ()  [unwired: 7 in, 3 out]
                  }
                  frame Enabled {
                  }
                }
                n347 = call-poly "Name to ref convert.vi"("name"="Waveform Chart") -> ("First REF"=w824:refnum<vi>)  [unwired: 10 in]
                n348 = call-poly "Name to ref convert.vi"("name"="Test Setting") -> ("First REF"=w813:refnum<vi>)  [unwired: 10 in]
                n349 = Build Array(w813) -> (w814:refnum<vi>[])
                n350 = To More Specific Class(target class=refnum<vi> refnum ("Waveform Chart"), reference=w824) -> (specific class reference=w822:refnum<vi>)  [unwired: 1 in, 1 out]
                n351 = property class="WFChart (strict)"(reference=w822, "History Data"=T28 []) -> ()  [unwired: 1 in, 2 out]
                n352 = call "Set Enable State on Multiple Controls.vi"("Enable?"=FALSE, "Controls"=w814) -> ()  [unwired: 9 in, 1 out]
                n353 = call-poly "Enqueue Message.vi"("Priority Message? (F)"=TRUE, "error in (no error)"=w826, "Message Data"=w817, "Message"="Start", "Message Queue"=w828) -> ("error out"=w829:errorcluster)  [unwired: 5 in, 1 out]
              }
            }
          }
          frame "Procedure Paused" {
            n354 = call-poly "Enqueue Message.vi"("Priority Message? (F)"=TRUE, "Message"="Step CW", "Message Queue"=w835) -> ()  [unwired: 7 in, 2 out]
            n355 = call-poly "Name to ref convert.vi"("name"="Stop Process") -> ("First REF"=w833:refnum<vi>)  [unwired: 10 in]
            n356 = property class="Ctl"(reference=w833, "Visible"=FALSE) -> ()  [unwired: 1 in, 2 out]
          }
        }
      }
      frame "Start Timer" {
        w845 = TRUE
        n357 = call-poly "Name to ref convert.vi"("name"="Timer Run") -> ("First REF"=w846:refnum<vi>)  [unwired: 10 in]
        n358 = call-poly "Name to ref convert.vi"("name"="Current Test") -> ("First REF"=w842:refnum<vi>)  [unwired: 10 in]
        n359 = call-poly "Name to ref convert.vi"("Array in"=string[] ["NEXT", "REDO"] ("name")) -> ("Array out"=w844:refnum<vi>[])  [unwired: 10 in]
        n360 = Build Array(w842) -> (w841:refnum<vi>[])
        n361 = property class="Ctl"(reference=w846, "Value"=w845, "Blinking"=w845) -> ()  [unwired: 1 in, 2 out]
        n362 = for {
          tunnel: w844 -> [w852] mode=indexing
          n363 = property class="Ctl"(reference=w852, "Visible"=FALSE) -> ()  [unwired: 1 in, 2 out]
        }
        n364 = call "Set Enable State on Multiple Controls.vi"("Enable?"=FALSE, "Controls"=w841) -> ()  [unwired: 9 in, 1 out]
      }
      frame "Start" {
        # "Start - Enable/Disable buttons appropriately for an acquisition that has started, and update status display."
        n365 = call-poly "Name to ref convert.vi"("Array in"=string[] ["Exit"]) -> ("Array out"=w856:refnum<vi>[])  [unwired: 10 in]
        n366 = call-poly "Name to ref convert.vi"("Array in"=string[] ["Save", "Test Setting", "Start Process", "Manual Switch"]) -> ("Array out"=w857:refnum<vi>[])  [unwired: 10 in]
        n367 = call "Set Enable State on Multiple Controls.vi"("Enable?"=FALSE, "Controls"=w856) -> ()  [unwired: 9 in, 1 out]
        n368 = call-poly "Enqueue Message.vi"("error in (no error)"=w863, "Message"="Init Modules", "Message Queue"=w864) -> ("error out"=w861:errorcluster)  [unwired: 7 in, 1 out]
        n369 = call "Set Enable State on Multiple Controls.vi"("Enable?"=TRUE, "Controls"=w857) -> ()  [unwired: 9 in, 1 out]
      }
      frame "Stop Process" {
        (unwired) "Stop Process" ("name")
        # "Start - Enable/Disable buttons appropriately for an acquisition that has started, and update status display."
        n370 = Unbundle By Name(w868) -> ("HIDEN"=w867:refnum<queue>)
        n371 = call "PCT Configure Enqueue CMD.vi"("Parameter Data"=TRUE ("Visible"), "CMD"=T4 {"Type CMD"="Mode", "Mode CMD"="", "Main CMD"="Action-Status"}, "CMD Queue in"=w877) -> ()  [unwired: 6 in, 3 out]
        n372 = call "FGV On Motion.vi"("CMD"=PCT_FGV_CMD."SET", "input"=FALSE) -> ()  [unwired: 8 in, 2 out]
        n373 = call-poly "Name to ref convert.vi"("name"="Stop Process") -> ("First REF"=w886:refnum<vi>)  [unwired: 10 in]
        n374 = call-poly "Name to ref convert.vi"("name"="Start Process") -> ("First REF"=w882:refnum<vi>)  [unwired: 10 in]
        n375 = call "PCT Configure Enqueue CMD.vi"("Priority Message? (F)"=TRUE, "CMD"=T4 {"Type CMD"="Stop Scan", "Mode CMD"="", "Main CMD"="Action-Status"}, "CMD Queue in"=w867) -> ()  [unwired: 6 in, 3 out]
        n376 = property class="Ctl"(reference=w886, "Visible"=FALSE) -> ()  [unwired: 1 in, 2 out]
        n377 = property class="Ctl"(reference=w882, "Value"=FALSE ("Visible")) -> ()  [unwired: 1 in, 2 out]
        n378 = call "Set Manual Tab Control Status.vi"("Value"=enum32{"Manual", "Test"}."Manual") -> ()  [unwired: 11 in]
        n379 = call-poly "Name to ref convert.vi"("name"="Test Setting") -> ("First REF"=w870:refnum<vi>)  [unwired: 10 in]
        n380 = Build Array(w870) -> (w871:refnum<vi>[])
        n381 = call "Set Enable State on Multiple Controls.vi"("Enable?"=TRUE, "Controls"=w871) -> ()  [unwired: 9 in, 1 out]
        n382 = call-poly "Name to ref convert.vi"("Array in"=string[] ["NEXT", "REDO"] ("name")) -> ("Array out"=w884:refnum<vi>[])  [unwired: 10 in]
        n383 = for {
          tunnel: w884 -> [w894] mode=indexing
          n384 = property class="Ctl"(reference=w894, "Visible"=FALSE) -> ()  [unwired: 1 in, 2 out]
        }
        n385 = call-poly "Enqueue Message.vi"("Priority Message? (F)"=TRUE, "Message"="Abort", "Message Queue"=w891) -> ("error out"=w892:errorcluster)  [unwired: 7 in, 1 out]
      }
      frame "Stop Timer" {
        w901 = FALSE
        n386 = call-poly "Name to ref convert.vi"("name"="Timer Run") -> ("First REF"=w902:refnum<vi>)  [unwired: 10 in]
        n387 = call-poly "Name to ref convert.vi"("Array in"=string[] ["NEXT", "REDO", "Current Test"] ("name")) -> ("Array out"=w900:refnum<vi>[])  [unwired: 10 in]
        n388 = Delete From Array(array=w900, length=1, index=2) -> (deleted portion=w898:refnum<vi>[], array with subset deleted=w899:refnum<vi>[])
        n389 = property class="Ctl"(reference=w902, "Value"=w901, "Blinking"=w901) -> ()  [unwired: 1 in, 2 out]
        n390 = for {
          tunnel: w899 -> [w909] mode=indexing
          n391 = property class="Ctl"(reference=w909, "Visible"=TRUE) -> ()  [unwired: 1 in, 2 out]
        }
        n392 = call "Set Enable State on Multiple Controls.vi"("Enable?"=TRUE, "Controls"=w898) -> ()  [unwired: 9 in, 1 out]
      }
      frame "Stop" {
        (unwired) "Test Setting" ("name")
        # "Stop - Enable/Disable buttons appropriately for an acquisition that has stopped, and update status display."
        n393 = call "Stop Modules.vi"("Message Queues in"=w914) -> ()  [unwired: 10 in, 1 out]
        n394 = call-poly "Name to ref convert.vi"("Array in"=string[] ["Exit"]) -> ("Array out"=w913:refnum<vi>[])  [unwired: 10 in]
        n395 = call "Set Enable State on Multiple Controls.vi"("Enable?"=TRUE, "Controls"=w913) -> ()  [unwired: 9 in, 1 out]
        n396 = call-poly "Name to ref convert.vi"("Array in"=string[] ["Save", "Start Process", "Manual Switch"]) -> ("Array out"=w915:refnum<vi>[])  [unwired: 10 in]
        n397 = Merge Errors(w919) -> (w920:errorcluster)
        n398 = call "Set Enable State on Multiple Controls.vi"("Enable?"=FALSE, "Controls"=w915) -> ()  [unwired: 9 in, 1 out]
      }
      frame "Switch Main Tab" {
        (unwired) enum16{"Test", "History"}."History" ("Tab Switch")
        (unwired) refnum<vi> refnum ("Main Tab")
        # "Start - Enable/Disable buttons appropriately for an acquisition that has started, and update status display."
        n399 = Variant To Data(type=FALSE ("x = y?"), Variant=w928) -> (data=w922:bool)  [unwired: 1 in, 1 out]
        n400 = call-poly "Name to ref convert.vi"("name"="Procedure Table") -> ("First REF"=w926:refnum<vi>)  [unwired: 10 in]
        n401 = call-poly "Name to ref convert.vi"("Array in"=string[] ["Report"] ("name")) -> ("Array out"=w924:refnum<vi>[])  [unwired: 10 in]
        n402 = call "Set Enable State on Multiple Controls.vi"("Enable?"=w922, "Controls"=w924) -> ()  [unwired: 9 in, 1 out]
        n403 = property class="Ctl"(reference=w926, "Visible"=w922) -> ()  [unwired: 1 in, 2 out]
      }
      frame "Update Status" {
        # "Update Status - Convert the message data to a string to display in the Status indicator."
        n404 = Variant To Data(error in=w945, type=T29 {"Message"="", "Message Data"=variant} ("Message Cluster"), Variant=w944) -> (data=w943:T29, error out=w936:errorcluster)
        n405 = Unbundle By Name(w943) -> ("Message"=w941:string, "Message Data"=w940:variant)
        n406 = case shown="\"Pump Status\"" w941 {
          selector: w941 -> [_ _ _ _ _ _ _ _ _ _ w1045 _ _ _ _ _ _ _]
          tunnel: w940 -> [_ _ w973 w984 w998 w1007 w1016 w1023 w1031 w1039 w1046 w1080 w1104 w1123 w1144 w1148 w1178 w1207]
          tunnel: w939 -> [w947 w953 w969 w981 w994 w1003 w1012 w1019 w1027 w1035 w1043 w1064 w1081 w1118 w1145 w1159 w1164 w1195]
          tunnel: [w947 w953 w969 w981 w994 w1003 w1012 w1019 w1027 w1035 w1047 w1064 w1081 w1118 w1145 w1159 w1164 w1195] -> w938
          tunnel: w937 -> [_ w964 _ _ _ _ _ _ _ _ _ _ _ _ _ _ _ _]
          tunnel: w935 -> [_ _ _ _ _ _ _ _ _ _ _ _ _ _ _ _ w1162 _]
          tunnel: w934 -> [_ _ _ w979 _ _ _ _ _ _ _ _ _ _ _ _ w1163 _]
          tunnel: w933 -> [w946 _ w968 w980 w993 w1002 w1011 w1018 w1026 w1034 w1042 w1076 w1100 w1119 w1142 w1146 w1161 w1191]
          tunnel: [w946 PCT_UI_State."Idle" ("UI State") w968 w980 w993 w1002 w1011 w1018 w1026 w1034 w1042 w1076 w1100 w1119 w1142 w1146 w1161 w1191] -> w932
          tunnel: w931 -> [_ _ _ _ _ _ _ _ _ _ _ _ _ _ _ _ w1160 _]
          frame "False", Default {
          }
          frame "Stop Process" {
            n407 = call-poly "Name to ref convert.vi"("name"="Start Process") -> ("First REF"=w966:refnum<vi>)  [unwired: 10 in]
            n408 = property class="Ctl"(reference=w966, "Value"=FALSE) -> ()  [unwired: 1 in, 2 out]
            n409 = call-poly "Name to ref convert.vi"("name"="XYZ Velocity") -> ("First REF"=w962:refnum<vi>)  [unwired: 10 in]
            n410 = call-poly "Name to ref convert.vi"("name"="Test Setting") -> ("First REF"=w949:refnum<vi>)  [unwired: 10 in]
            n411 = call "Set Manual Tab Control Status.vi"("Value"=enum32{"Manual", "Test"}."Manual") -> ()  [unwired: 11 in]
            n412 = property class="Ctl"(reference=w962) -> ("Value"=w960:variant)  [unwired: 1 in, 2 out]
            n413 = Build Array(w949) -> (w950:refnum<vi>[])
            n414 = call-poly "Name to ref convert.vi"("name"="Stop Process") -> ("First REF"=w955:refnum<vi>)  [unwired: 10 in]
            n415 = call "Set Enable State on Multiple Controls.vi"("Enable?"=TRUE, "Controls"=w950) -> ()  [unwired: 9 in, 1 out]
            n416 = Variant To Data(type=u16 50 ("SET VEL"), Variant=w960) -> (data=w954:u16)  [unwired: 1 in, 1 out]
            n417 = property class="Ctl"(reference=w955, "Visible"=FALSE) -> ()  [unwired: 1 in, 2 out]
            n418 = call-poly "Enqueue Message.vi"("Message Data"=w954, "Message"="Manual SET VEL", "Message Queue"=w964) -> ()  [unwired: 7 in, 2 out]
          }
          frame "DB Status" {
            n419 = Variant To Data(type=FALSE, Variant=w973) -> (data=w971:bool)  [unwired: 1 in, 1 out]
            n420 = call-poly "Name to ref convert.vi"("name"="DB") -> ("First REF"=w974:refnum<vi>)  [unwired: 10 in]
            n421 = Not(x=w971) -> (.not. x?=w970:bool)
            n422 = property class="Ctl"(reference=w974, "Value"=w970) -> ()  [unwired: 1 in, 2 out]
          }
          frame "HIDEN Status" {
            n423 = Variant To Data(type=FALSE, Variant=w984) -> (data=w982:bool)  [unwired: 1 in, 1 out]
            n424 = Unbundle By Name(w979) -> ("HIDEN"=w978:refnum<queue>)
            n425 = call-poly "Name to ref convert.vi"("name"="Hiden Status") -> ("First REF"=w985:refnum<vi>)  [unwired: 10 in]
            n426 = Not(x=w982) -> (.not. x?=w977:bool)
            n427 = property class="Ctl"(reference=w985, "Value"=w977) -> ()  [unwired: 1 in, 2 out]
            n428 = case shown="True" FALSE {
              tunnel: w978 -> [_ w987]
              frame False {
              }
              frame True {
                n429 = call "PCT Configure Enqueue CMD.vi"("Parameter Data"=0, "CMD"=T4 {"Type CMD"="Start Scan", "Mode CMD"="", "Main CMD"="Action-Status"}, "CMD Queue in"=w987) -> ("error out"=w992:errorcluster, "CMD Queue out"=w991:refnum<queue>)  [unwired: 6 in, 1 out]
                n430 = call "PCT Configure Enqueue CMD.vi"("error in (no error)"=w992, "CMD"=T4 {"Type CMD"="", "Mode CMD"="", "Main CMD"="Data"}, "CMD Queue in"=w991) -> ()  [unwired: 6 in, 3 out]
              }
            }
          }
          frame "PalmSense Status" {
            n431 = Variant To Data(type=FALSE, Variant=w998) -> (data=w996:bool)  [unwired: 1 in, 1 out]
            n432 = Not(x=w996) -> (.not. x?=w995:bool)
            n433 = call-poly "Name to ref convert.vi"("name"="PS Status") -> ("First REF"=w999:refnum<vi>)  [unwired: 10 in]
            n434 = property class="Ctl"(reference=w999, "Value"=w995) -> ()  [unwired: 1 in, 2 out]
          }
          frame "Motor Status" {
            n435 = call "Set Manual Tab Control Status.vi"("Value"=enum32{"Manual", "Test"}."Manual") -> ()  [unwired: 11 in]
            n436 = Variant To Data(type=FALSE, Variant=w1007) -> (data=w1005:bool)  [unwired: 1 in, 1 out]
            n437 = call-poly "Name to ref convert.vi"("name"="Motor Status") -> ("First REF"=w1008:refnum<vi>)  [unwired: 10 in]
            n438 = Not(x=w1005) -> (.not. x?=w1004:bool)
            n439 = property class="Ctl"(reference=w1008, "Value"=w1004) -> ()  [unwired: 1 in, 2 out]
          }
          frame "Pump Status" {
            n440 = Variant To Data(type=FALSE, Variant=w1016) -> (data=w1014:bool)  [unwired: 1 in, 1 out]
            n441 = call-poly "Name to ref convert.vi"("name"="Pump Status") -> ("First REF"=w1017:refnum<vi>)  [unwired: 10 in]
            n442 = Not(x=w1014) -> (.not. x?=w1013:bool)
            n443 = property class="Ctl"(reference=w1017, "Value"=w1013) -> ()  [unwired: 1 in, 2 out]
          }
          frame "SYS 7000 Reader" {
            n444 = Variant To Data(type=FALSE, Variant=w1023) -> (data=w1021:bool)  [unwired: 1 in, 1 out]
            n445 = call-poly "Name to ref convert.vi"("name"="SYS 7000 Reader") -> ("First REF"=w1024:refnum<vi>)  [unwired: 10 in]
            n446 = Not(x=w1021) -> (.not. x?=w1020:bool)
            n447 = property class="Ctl"(reference=w1024, "Value"=w1020) -> ()  [unwired: 1 in, 2 out]
          }
          frame "PS Status" {
            n448 = Variant To Data(type=FALSE, Variant=w1031) -> (data=w1029:bool)  [unwired: 1 in, 1 out]
            n449 = call-poly "Name to ref convert.vi"("name"="PS Status") -> ("First REF"=w1032:refnum<vi>)  [unwired: 10 in]
            n450 = Not(x=w1029) -> (.not. x?=w1028:bool)
            n451 = property class="Ctl"(reference=w1032, "Value"=w1028) -> ()  [unwired: 1 in, 2 out]
          }
          frame "MFC Status" {
            n452 = Variant To Data(type=FALSE, Variant=w1039) -> (data=w1037:bool)  [unwired: 1 in, 1 out]
            n453 = call-poly "Name to ref convert.vi"("name"="MFC Status") -> ("First REF"=w1040:refnum<vi>)  [unwired: 10 in]
            n454 = Not(x=w1037) -> (.not. x?=w1036:bool)
            n455 = property class="Ctl"(reference=w1040, "Value"=w1036) -> ()  [unwired: 1 in, 2 out]
          }
          frame "Test Date Update" {
            n456 = Variant To Data(type=w1045, Variant=w1046) -> (data=w1044:string)  [unwired: 1 in, 1 out]
            n457 = Bundle By Name(cluster=w1043, "Report Configuration.Test Setting.Date"=w1044) -> (w1047:T7)
          }
          frame "Update Procedure" {
            n458 = Variant To Data(type=dbl[] [] ("Current SP"), Variant=w1080) -> (data=w1070:dbl[])  [unwired: 1 in, 1 out]
            n459 = call "FGV GAGE Zero.vi"("CMD"=PCT_FGV_CMD."GET") -> ("output"=w1050:dbl[])  [unwired: 9 in, 1 out]
            n460 = Unbundle By Name(w1064) -> ("Process.Test Configuration.System Preset.Test Configuration.SP List"=w1060:dbl[][])
            n461 = Array To Cluster(array=w1070) -> (cluster=w1063:T34)
            n462 = Index Array(array=w1050) -> (element=w1049:dbl)  [unwired: 1 in]
            n463 = call-poly "Name to ref convert.vi"("name"="SP List Ind") -> ("First REF"=w1077:refnum<vi>)  [unwired: 10 in]
            n464 = Unbundle(w1063) -> ("Current SP[0]"=w1048:dbl, "Current SP[1]"=w1062:dbl)
            n465 = call-poly "Name to ref convert.vi"("name"="XY Graph") -> ("First REF"=w1072:refnum<vi>)  [unwired: 10 in]
            n466 = Index Array(array=w1070, index=2) -> (element=w1066:dbl)
            n467 = Index Array(array=w1060, index (col) #1=0 ("disabled index (col)"), index (col) #2=1 ("index (col)")) -> (element #1=w1057:dbl[], element #2=w1055:dbl[])  [unwired: 2 in]
            n468 = Subtract(x=w1049, y=w1048) -> ()  [unwired: 1 out]
            n469 = Equal To 0?(x=w1066) -> (x = 0?=w1065:bool)
            n470 = call "Convert to Dynamic Data"("Array"=w1057) -> ("Dynamic Data Type"=w1056:dynamicdata)  [unwired: 3 in]
            n471 = call "Convert to Dynamic Data2"("Array"=w1055) -> ("Dynamic Data Type"=w1054:dynamicdata)  [unwired: 3 in]
            n472 = To More Specific Class(target class=refnum<vi> refnum ("XY Graph"), reference=w1072) -> (specific class reference=w1071:refnum<vi>)  [unwired: 1 in, 1 out]
            n473 = To More Specific Class(target class=refnum<vi> refnum ("SP List Ind"), reference=w1077) -> (specific class reference=w1074:refnum<vi>)  [unwired: 1 in, 1 out]
            n474 = call "Build XY Graph"("Reset"=w1065, "Y Input"=w1062, "X Input"=w1048) -> ("XY Graph"=w1061:cluster{"X":dbl[], "Y":dbl[]}[])  [unwired: 7 in, 1 out]
            n475 = call "Build XY Graph4"("Reset"=TRUE, "Y Input"=w1054, "X Input"=w1056) -> ("XY Graph"=w1053:cluster{"X":dbl[], "Y":dbl[]}[])  [unwired: 7 in, 1 out]
            n476 = property class="MCListbox (strict)"(reference=w1074, "Value"=w1066) -> ()  [unwired: 1 in, 2 out]
            n477 = Build Array (concatenate)(w1061, w1053) -> (w1069:cluster{"X":dbl[], "Y":dbl[]}[])
            n478 = property class="XYGraph (strict)"(reference=w1071, "Value"=w1069) -> ()  [unwired: 1 in, 2 out]
          }
          frame "Update XY Graph" {
            n479 = Variant To Data(type=dbl[] [] ("Current SP"), Variant=w1104) -> (data=w1094:dbl[])  [unwired: 1 in, 1 out]
            n480 = call "FGV GAGE Zero.vi"("CMD"=PCT_FGV_CMD."GET") -> ("output"=w1084:dbl[])  [unwired: 9 in, 1 out]
            n481 = Array To Cluster(array=w1094) -> (cluster=w1088:T34)
            n482 = Index Array(array=w1084) -> (element=w1083:dbl)  [unwired: 1 in]
            n483 = call-poly "Name to ref convert.vi"("name"="SP List Ind") -> ("First REF"=w1101:refnum<vi>)  [unwired: 10 in]
            n484 = Unbundle(w1088) -> ("Current SP[0]"=w1082:dbl, "Current SP[1]"=w1087:dbl)
            n485 = call-poly "Name to ref convert.vi"("name"="XY Graph") -> ("First REF"=w1096:refnum<vi>)  [unwired: 10 in]
            n486 = Index Array(array=w1094, index=2) -> (element=w1090:dbl)
            n487 = Subtract(x=w1083, y=w1082) -> ()  [unwired: 1 out]
            n488 = Equal To 0?(x=w1090) -> (x = 0?=w1089:bool)
            n489 = To More Specific Class(target class=refnum<vi> refnum ("XY Graph"), reference=w1096) -> (specific class reference=w1095:refnum<vi>)  [unwired: 1 in, 1 out]
            n490 = To More Specific Class(target class=refnum<vi> refnum ("SP List Ind"), reference=w1101) -> (specific class reference=w1098:refnum<vi>)  [unwired: 1 in, 1 out]
            n491 = call "Build XY Graph5"("Reset"=w1089, "Y Input"=w1087, "X Input"=w1082) -> ("XY Graph"=w1086:cluster{"X":dbl[], "Y":dbl[]}[])  [unwired: 7 in, 1 out]
            n492 = property class="MCListbox (strict)"(reference=w1098, "Value"=w1090) -> ()  [unwired: 1 in, 2 out]
            n493 = Build Array (concatenate)(w1086) -> (w1093:cluster{"X":dbl[], "Y":dbl[]}[])
            n494 = property class="XYGraph (strict)"(reference=w1095, "Value"=w1093) -> ()  [unwired: 1 in, 2 out]
          }
          frame "Reset XY Graph" {
            n495 = Variant To Data(type=i32[] [] ("Current SP"), Variant=w1123) -> (data=w1111:i32[])  [unwired: 1 in, 1 out]
            n496 = Index Array(array=w1111) -> (element=w1115:i32)  [unwired: 1 in]
            n497 = Array To Cluster(array=w1111) -> (cluster=w1110:T35)
            n498 = call-poly "Name to ref convert.vi"("name"="SP List Ind") -> ("First REF"=w1120:refnum<vi>)  [unwired: 10 in]
            n499 = Unbundle(w1110) -> ("Current SP[0]"=w1109:i32, "Current SP[1]"=w1108:i32)
            n500 = call-poly "Name to ref convert.vi"("name"="XY Graph") -> ("First REF"=w1113:refnum<vi>)  [unwired: 10 in]
            n501 = call "Build XY Graph2"("Reset"=FALSE, "Y Input"=w1108, "X Input"=w1109) -> ("XY Graph"=w1107:cluster{"X":dbl[], "Y":dbl[]}[])  [unwired: 7 in, 1 out]
            n502 = To More Specific Class(target class=refnum<vi> refnum ("XY Graph"), reference=w1113) -> (specific class reference=w1112:refnum<vi>)  [unwired: 1 in, 1 out]
            n503 = To More Specific Class(target class=refnum<vi> refnum ("SP List Ind"), reference=w1120) -> (specific class reference=w1116:refnum<vi>)  [unwired: 1 in, 1 out]
            n504 = property class="MCListbox (strict)"(reference=w1116, "Value"=w1115) -> ()  [unwired: 1 in, 2 out]
            n505 = property class="XYGraph (strict)"(reference=w1112, "Value"=w1107) -> ()  [unwired: 1 in, 2 out]
          }
          frame "Update RES Table" {
            n506 = Variant To Data(type=string[] [] ("Array"), Variant=w1144) -> (data=w1141:string[])  [unwired: 1 in, 1 out]
            n507 = Delete From Array(array=w1141, length=1, index=0) -> (deleted portion=w1138:string[])  [unwired: 1 out]
            n508 = call-poly "Name to ref convert.vi"("name"="Test Step Done") -> ("First REF"=w1135:refnum<vi>)  [unwired: 10 in]
            n509 = To More Specific Class(target class=refnum<vi> refnum ("Test Step Done"), reference=w1135) -> (specific class reference=w1134:refnum<vi>, error out=w1133:errorcluster)  [unwired: 1 in]
            n510 = Index Array(array=w1138, index=0) -> (element=w1130:string)
            n511 = property class="MCListbox (strict)"(reference=w1134, error in=w1133) -> (reference out=w1128:refnum<vi>, "ItemNames"=w1131:string[][])  [unwired: 1 out]
            n512 = Build Array(w1130, "DONE" ("element")) -> (w1129:string[])
            n513 = Build Array (concatenate)(w1131, w1129) -> (w1127:string[][])
            n514 = property class="MCListbox (strict)"(reference=w1128, "ItemNames"=w1127, "ActiveCell"=T30 {"Row"=0, "Column"=0} ("Active Cell:Active Cell"), "CellFontColor"=u32 0) -> ()  [unwired: 1 in, 2 out]
          }
          frame "Update Limit Table" {
            n515 = Variant To Data(type=T31 {"Writer Queue"=refnum, "Writer Data"={"Message"="", "Message Data"=variant}} ("HW Message"), Variant=w1148) -> (data=w1149:T31)  [unwired: 1 in, 1 out]
            n516 = Unbundle By Name(w1149) -> ("Writer Data.Message Data"=w1147:variant)  [unwired: 1 out]
            n517 = Variant To Data(type=dbl[][] [] ("Row Limit"), Variant=w1147) -> (data=w1153:dbl[][])  [unwired: 1 in, 1 out]
            n518 = call-poly "Name to ref convert.vi"("name"="Step Limit Table") -> ("First REF"=w1158:refnum<vi>)  [unwired: 10 in]
            n519 = To More Specific Class(target class=refnum<vi> refnum ("Limit Table"), reference=w1158) -> (specific class reference=w1157:refnum<vi>)  [unwired: 1 in, 1 out]
            n520 = Number To Fractional String(number=w1153, precision (6)=i16 1) -> (F-format string=w1151:string[][])  [unwired: 2 in]
            n521 = property class="Tbl (strict)"(reference=w1157, "Value"=w1151) -> ()  [unwired: 1 in, 2 out]
          }
          frame "PLC Error" {
            n522 = disable-structure shown="Enabled" {
              disable-tunnel: w1163 -> [w1186 w1188]
              disable-tunnel: w1162 -> [w1184 _]
              disable-tunnel: w1160 -> [_ _]
              frame Disabled {
                n523 = Unbundle By Name(w1184) -> ("Motor notifier"=w1183:refnum<notifier>)
                n524 = Unbundle By Name(w1186) -> ("Logging"=w1185:refnum<queue>, "VALVE"=w1180:refnum<queue>)
                n525 = Get Notifier Status(notifier=w1183) -> (current notification=w1179:i32)  [unwired: 1 in, 4 out]
                n526 = Number To Decimal String(number=w1179) -> (decimal integer string=w1181:string)  [unwired: 1 in]
                n527 = call-poly "Enqueue Message.vi"("Message Data"=w1181, "Message"="Acquire", "Message Queue"=w1180) -> ()  [unwired: 7 in, 2 out]
                n528 = call-poly "Enqueue Message.vi"("Message Data"=w1179, "Message"="Log", "Message Queue"=w1185) -> ()  [unwired: 7 in, 2 out]
              }
              frame Enabled {
                n529 = disable-structure shown="Disabled" {
                  disable-tunnel: w1188 -> [w1190 _]
                  frame Disabled {
                    n530 = call "AM Stopping Procedure.vi"("Stop"=FALSE ("Priority Message? (F)"), "Message Queues in"=w1190) -> ()  [unwired: 9 in, 1 out]
                  }
                  frame Enabled {
                  }
                }
              }
            }
            n531 = Variant To Data(type=errorcluster {"status"=FALSE, "code"=0, "source"=""} ("error out"), Variant=w1178) -> (data=w1176:errorcluster)  [unwired: 1 in, 1 out]
            n532 = Unbundle By Name(w1176) -> ("code"=w1170:i32)
            n533 = Subtract(x=w1170, y=5100) -> (x-y=w1167:i32)
            n534 = call-poly "Name to ref convert.vi"("Array in"=string[] ["Reset Error", "Alarm Display"] ("name")) -> ("Array out"=w1173:refnum<vi>[])  [unwired: 10 in]
            n535 = Number To Decimal String(number=w1167) -> (decimal integer string=w1166:string)  [unwired: 1 in]
            n536 = Index Array(array=w1173) -> (element #1=w1174:refnum<vi>, element #2=w1172:refnum<vi>)  [unwired: 2 in]
            n537 = Not Equal To 0?(x=w1167) -> (x != 0?=w1168:bool)
            n538 = call "FGV ALL Alarms.vi"("CMD"=PCT_FGV_CMD."GET", "name"=w1166) -> ("Alarm MSG out"=w1165:string)  [unwired: 8 in, 1 out]
            n539 = property class="Ctl"(reference=w1174, "Visible"=w1168) -> ()  [unwired: 1 in, 2 out]
            n540 = property class="Ctl"(reference=w1172, "Visible"=w1168, "Value"=w1165) -> ()  [unwired: 1 in, 2 out]
          }
          frame "Test Step CW" {
            n541 = Variant To Data(type=cluster{"current Step":i32, "Data to Res":dbl[]} {"current Step"=0, "Data to Res"=[]} ("output cluster"), Variant=w1207) -> (data=w1201:cluster{"current Step":i32, "Data to Res":dbl[]})  [unwired: 1 in, 1 out]
            n542 = Unbundle By Name(w1201) -> ("current Step"=w1200:i32, "Data to Res"=w1199:dbl[])
            n543 = call-poly "Name to ref convert.vi"("name"="Results") -> ("First REF"=w1205:refnum<vi>)  [unwired: 10 in]
            n544 = Type Cast(type=refnum<vi> refnum ("Results"), x=w1205) -> (*(type *) &x=w1197:refnum<vi>)
            n545 = Number To Fractional String(number=w1199, precision (6)=i16 1) -> (F-format string=w1198:string[])  [unwired: 2 in]
            n546 = property class="Tbl (strict)"(reference=w1197) -> (reference out=w1203:refnum<vi>, "Value"=w1202:string[][])  [unwired: 1 in, 1 out]
            n547 = Replace Array Subset(array=w1202, new element=w1198, index (row)=w1200) -> (w1194:string[][])  [unwired: 1 in]
            n548 = property class="Tbl (strict)"(reference=w1203, "Value"=w1194) -> (reference out=w1196:refnum<vi>)  [unwired: 1 in, 1 out]
            n549 = call "RES Get Max value.vi"("Table in"=w1196) -> ()  [unwired: 11 in]
          }
        }
      }
      frame "Valve Response" {
        # "Start - Enable/Disable buttons appropriately for an acquisition that has started, and update status display."
        n550 = Variant To Data(type=bool[] [FALSE, FALSE] ("FixElevationValve"), Variant=w1213) -> (data=w1211:bool[])  [unwired: 1 in, 1 out]
        n551 = Not(x=w1211) -> (.not. x?=w1210:bool[])
        n552 = And Array Elements(Boolean array=w1210) -> (logical AND=w1209:bool)
        n553 = call-poly "Name to ref convert.vi"("Array in"=string[] ["FixActuatorsValve", "Set Valves"] ("name")) -> ("Array out"=w1219:refnum<vi>[])  [unwired: 10 in]
        n554 = Not(x=w1209) -> (.not. x?=w1208:bool)
        n555 = Index Array(array=w1219) -> (element #1=w1217:refnum<vi>, element #2=w1215:refnum<vi>)  [unwired: 2 in]
        n556 = To More Specific Class(target class=refnum<vi> refnum ("FixActuatorsValve"), reference=w1217) -> (specific class reference=w1218:refnum<vi>)  [unwired: 1 in, 1 out]
        n557 = property class="Arr (strict)"(reference=w1218, "Value"=w1211) -> ()  [unwired: 1 in, 2 out]
        n558 = property class="Ctl"(reference=w1215, "Value"=w1208) -> ()  [unwired: 1 in, 2 out]
      }
      frame Default {
        # "'Default' case only runs if there is a message that isn't defined in any of the other cases.  Output a programming error."
        n559 = xnode "Error Ring"("parameter 0"=w1225) -> ("error out"=w1224:errorcluster)
      }
    }
    n560 = call "Error Handler - Message Handling Loop.vi"("error in (no error)"=w25, "Message Queue"=w20) -> ("dup error in"=w26:errorcluster)  [unwired: 8 in, 1 out]
  }
  "error out" <- w14
